vi "Marvin.vi"() -> ()   [LabVIEW 2017]
uses:
  Marvin ATP Remake 1.5.18/PCAN_Driver/ControlCAN.llb/CAN Channel.ctl
  Marvin ATP Remake 6.5.18 - Copy/PCAN_Driver/ControlCAN.llb/DevType.ctl
  Marvin ATP Remake 6.5.18/PCAN_Driver/ControlCAN.llb/VCI_INIT_CONFIG.ctl
  Marvin ATP Remake 6.5.18/PCAN_Driver/ControlCAN.llb/InitFlag.ctl
  Marvin ATP Remake 6.5.18/PCAN_Driver/ControlCAN.llb/Fliter.ctl
  Marvin ATP Remake 6.5.18/PCAN_Driver/ControlCAN.llb/Mode.ctl
  <vilib>/Utility/miscctls.llb/LVMinMaxIncTypeDef.ctl
  PCAN_Driver/ControlCAN.llb/VCI_CAN_OBJ.ctl
  PCAN_Driver/ControlCAN.lvlib
panel:
  in  "Clear Data Array":bool
  in  "PlayPause Data Array":bool
  out "CAN Data":cluster{"Frame Data":u64, "Frame ID":u32}[](array[cluster]) {"Frame ID" format="%.0x"; "Frame Data" format="%016x"}
  out "Waveform Chart":dbl[](graph)
  in  "Help Button":bool
  in  "Clear Monitor":bool
  out "Array":u64[][](array[numeric]) format="%016x"
  out "Ambient Over temp":bool
  out "Ambient Sensor temp":bool
  out "Ambient Temperature":dbl
  in  "Motor Over Temp":bool
  in  "Speed control":bool
  out "Unit Adress":string
  in  "Serial Send":bool
  in  "Index":u16(ring) items=["1"=1, "2"=2, "3"=3]
  out "read buffer":string
  in  "SetGet":enum16{"Get", "Set"}(ring)
  in  "Function":T1(ring)
  in  "Value":dbl
  in  "Value 1/2":enum16{"1", "2"}(ring)
  out "Msg Count":u32
  in  "Param to Set":u16(ring) items=["EBAY 5F"=95, "AHU 3F"=63, "AHU 2F"=47]
  out "UUT":u8
  out "Horizontal Progress Bar":i32(slide) min=0 max=48 scale=0.0..50.0
  in  "Set Param.":bool
  in  "Serial Monitor":bool caption="Graph Button"
  in  "Serial Com":bool
  in  "VISA resource name":refnum<visa-resource-name>="COM6"
  out "Serial Status":bool
  in  "Graph Button":bool
  in  "Refresh Button":bool
  out "Data Send":u64 format="%016x"
  in  "Motor Speed RPM":u16
  out "Under voltage/Over voltage":bool
  out "Speed error":bool
  out "Derated drive temp":bool
  out "Motor Over temperature":bool
  out "Commutation err":bool
  out "Motor Sensor temp Fauilre":bool
  out "Drive Over temperature":bool
  out "Drive Sensor temp Failure":bool
  out "Motor Phase Current RMS":dbl
  out "ECS State":u16
  out "Motor Speed RPM":dbl
  out "Motor Stator Temp.":dbl
  out "Power transistor Heat sink Temp.":dbl
  out "DC Current":dbl
  out "DC Voltage":dbl
  in  "Can Send":bool
  in  "Stop":bool
  out "Config_CANAT":T8 {"DevType" items=["USB-CAN"=3, "USB-CAN2"=4]; "CanIndex" items=["通道1", "通道2"]; "VCI_INIT_CONFIG"."Fliter" items=["接收所有类型"=3, "只接收标准帧"=4, "只接收扩展帧"=7]; "VCI_INIT_CONFIG"."Mode" items=["正常工作", "自测模式（环回）", "仅侦听模式"]; "VCI_INIT_CONFIG"."InitFlag" items=["使用Flash参数", "使用界面设置参数"]}
  in  "Channel 2":T3 caption="Channel" items=["Channel 1", "Channel 2"]
  out "CAN Status":bool
  out "Driver Version":string
  out "Hall Sensor Fault":bool
  out "Motor Phase Current":u16
  in  "Motor Phase Current":u16
  # "ver 1.7"
  # "Marvin"
  # "REDLER TECHNOLOGIES LTD"
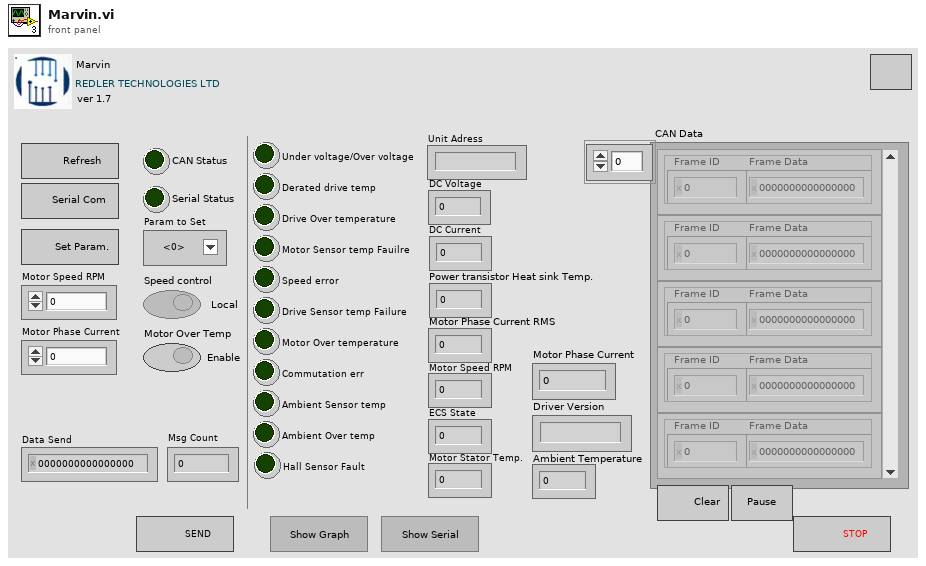
[diagram p1: front panel]
types:
  T1 = enum16{"Enable Conf. EP=1", "Serial Number", "Temperature", "Unit Adress", "Calibration", "Velocity", "Version"}
  T2 = typedef "ControlCAN.lvlib/DevType.ctl" = u32
  T3 = typedef "ControlCAN.lvlib/CAN Channel.ctl" = u32
  T4 = typedef "ControlCAN.lvlib/VCI_INIT_CONFIG.ctl" = cluster{"AccCode":u32, "AccMask":u32, "InitFlag":T5, "Fliter":T6, "Timing0":u8, "Timing1":u8, "Mode":T7}
  T5 = typedef "ControlCAN.lvlib/InitFlag.ctl" = u32
  T6 = typedef "ControlCAN.lvlib/Fliter.ctl" = u8
  T7 = typedef "ControlCAN.lvlib/Mode.ctl" = u8
  T8 = cluster{"DevType":T2, "DevIndex":u32, "CanIndex":T3, "VCI_INIT_CONFIG":T4}
  T9 = cluster{"ID":u32, "MSGTYPE":u8, "LEN":u8, "aDATA":u8[]}[]
  T10 = cluster{"ID":u32, "MSGTYPE":u8, "LEN":u8, "aDATA":u8[]}
  T11 = enum8{"Enabled", "Disabled", "Disabled and Grayed Out"}
  T12 = typedef "LVMinMaxIncTypeDef.ctl" = cluster{"Minimum":dbl, "Maximum":dbl, "Increment":dbl}
  T13 = enum32{"Invalid", "Standard", "Closed", "Hidden", "Minimized", "Maximized"}
  T14 = typedef "ControlCAN.lvlib/VCI_CAN_OBJ.ctl" = cluster{"ID":u32, "TimeStamp":u32, "TimeFlag":u8, "SendType":u8, "RemoteFlag":u8, "ExternFlag":u8, "DataLen":u8, "Data":u8[], "Reserved":u8[]}
  T15 = cluster{"Type":enum16{"接收", "发送"}, "Channel":T3, "Time":timestamp, "VCI_CAN_OBJ":T14}[]
  T16 = cluster{"Type":enum16{"接收", "发送"}, "Channel":T3, "Time":timestamp, "VCI_CAN_OBJ":T14}
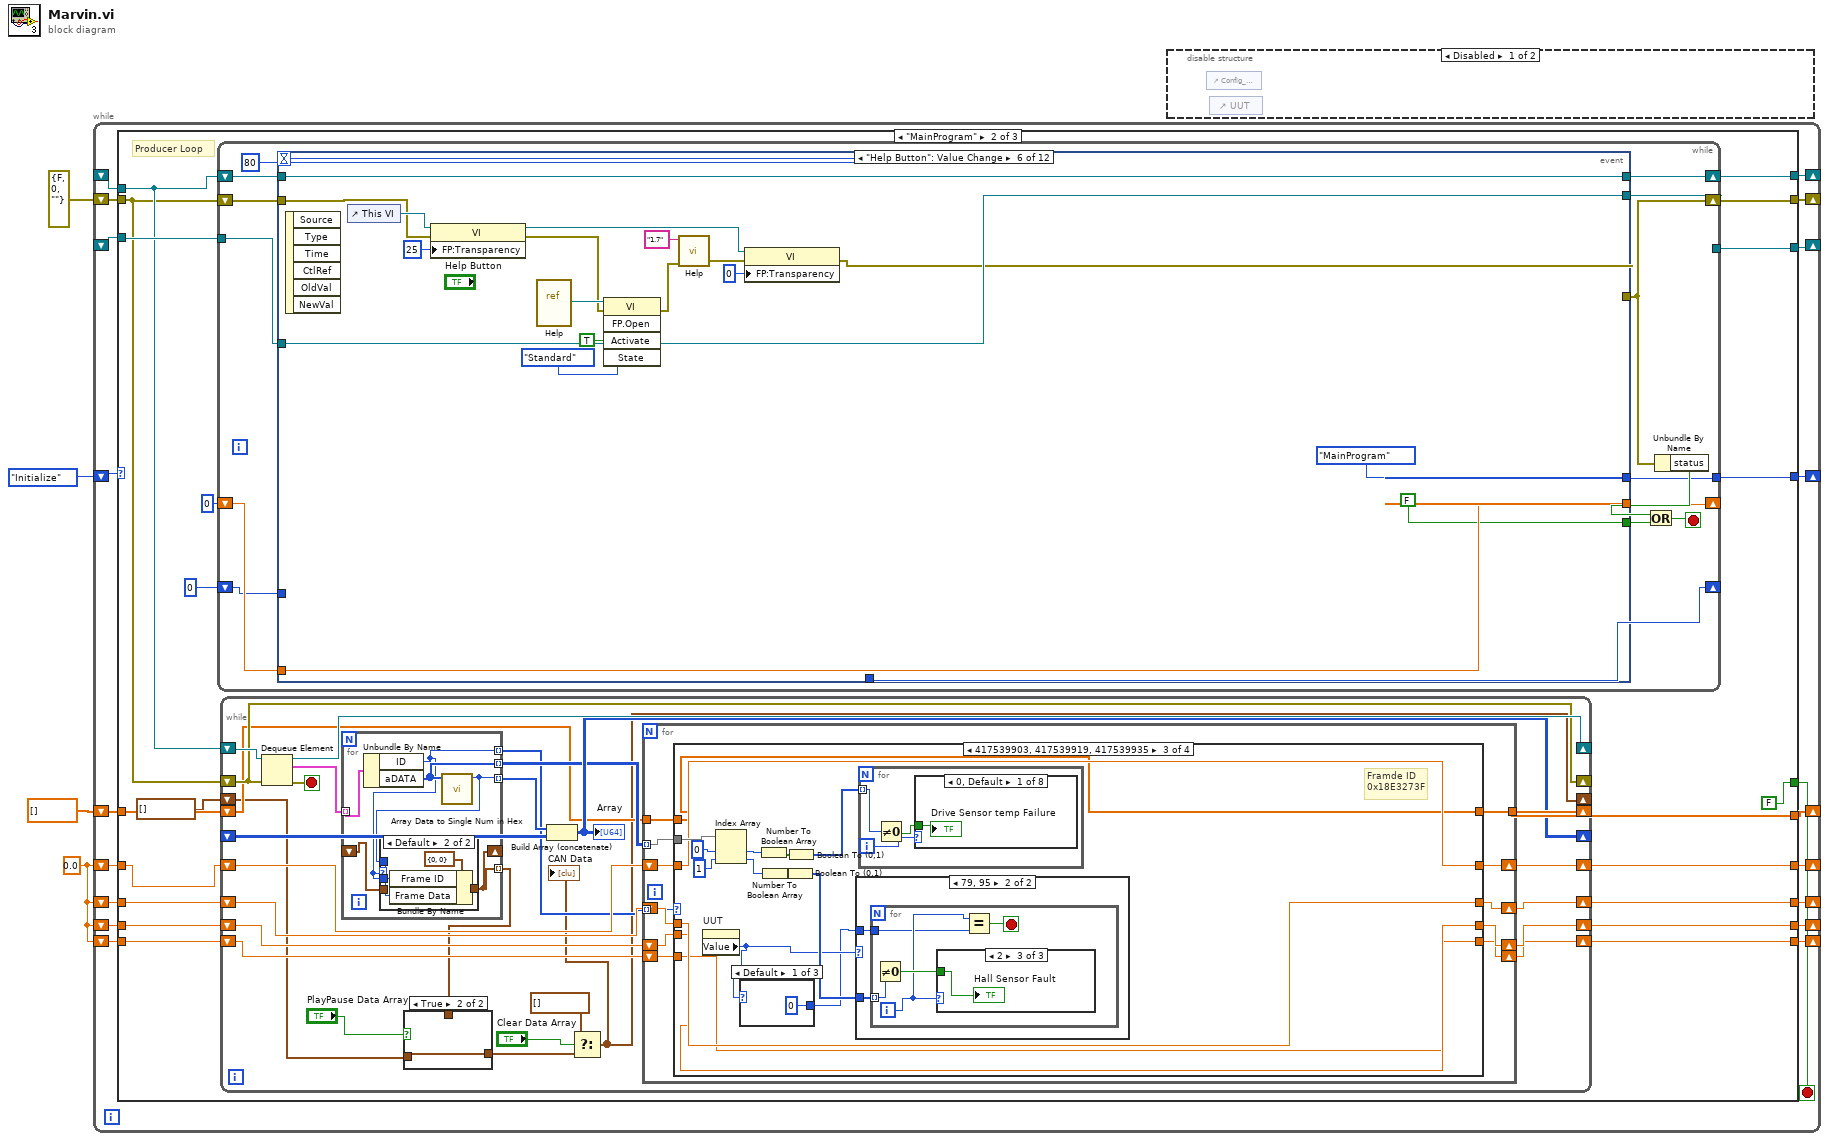
[diagram p0: block diagram]
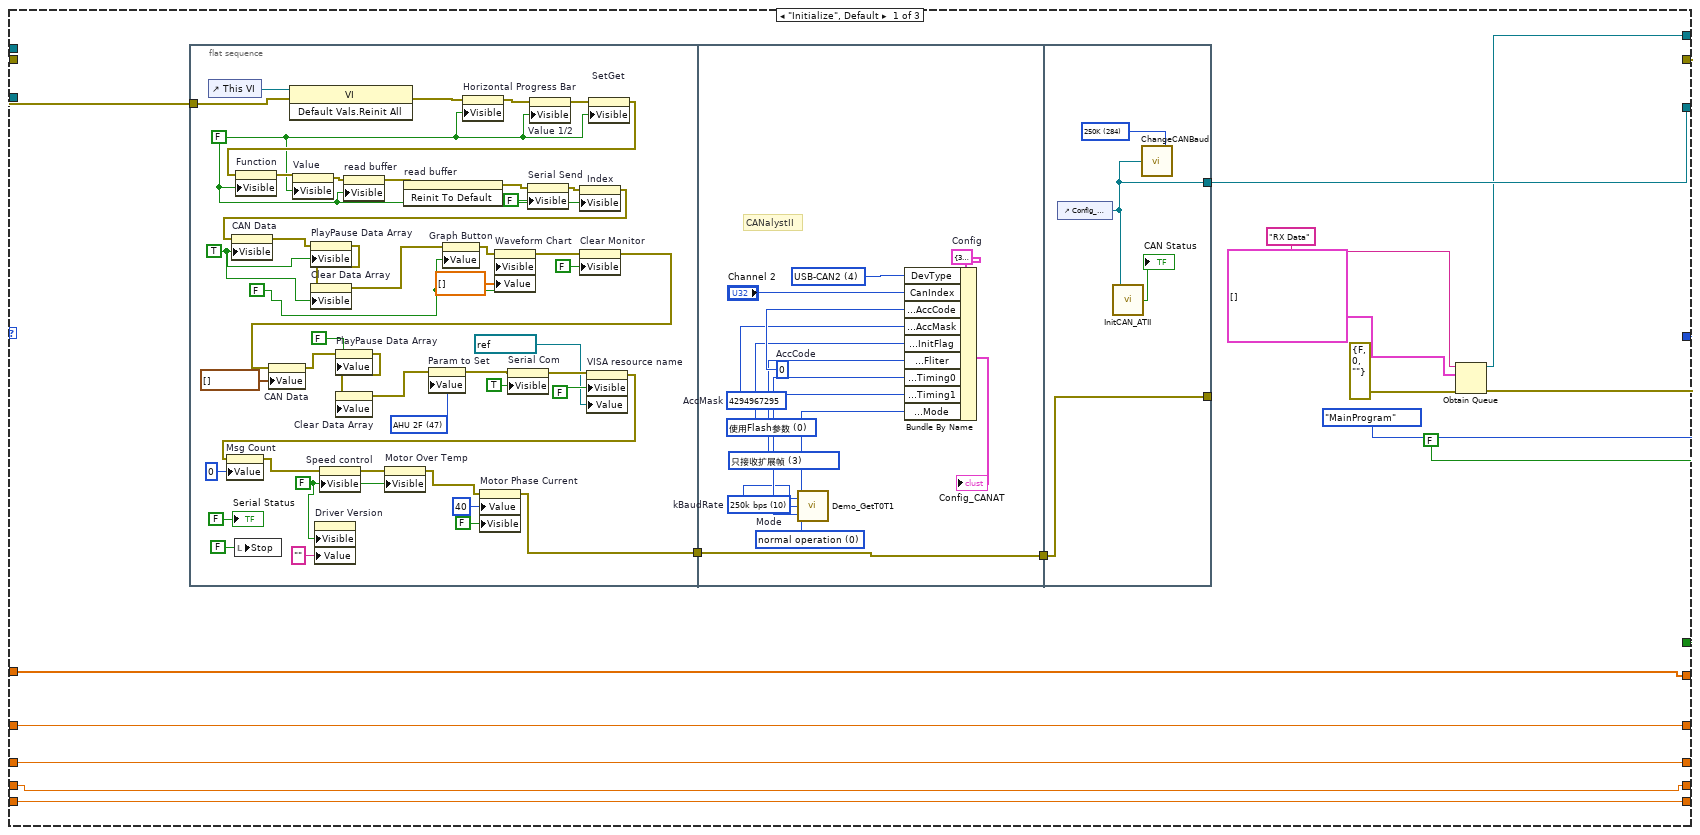
[diagram p3: hidden frame]
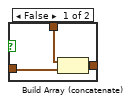
[diagram p4: hidden frame]
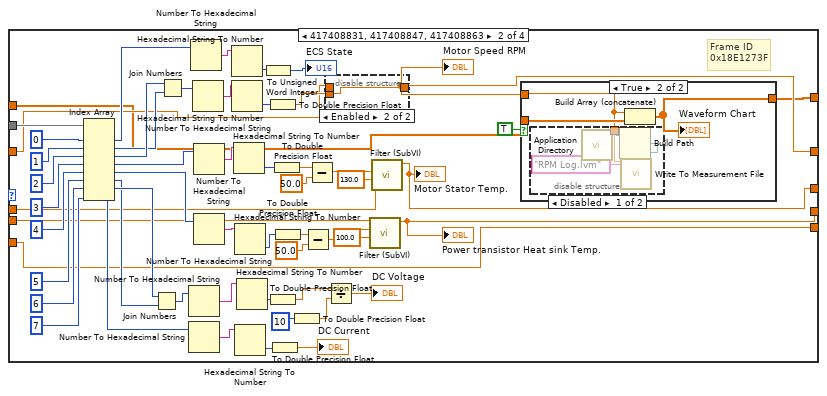
[diagram p6: hidden frame]
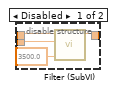
[diagram p7: hidden frame]
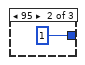
[diagram p10: hidden frame]
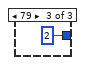
[diagram p11: hidden frame]
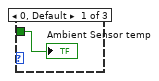
[diagram p13: hidden frame]
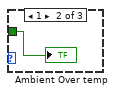
[diagram p14: hidden frame]
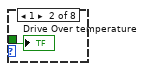
[diagram p15: hidden frame]
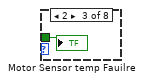
[diagram p16: hidden frame]
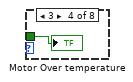
[diagram p17: hidden frame]
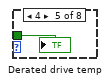
[diagram p18: hidden frame]
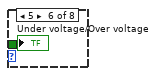
[diagram p19: hidden frame]
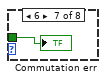
[diagram p20: hidden frame]
diagram:
  w2 = 0.0
  n1 = while {
    shift-right: [w18] -> _
    shift-left: enum16{"Stop", "MainProgram", "Initialize"}."Initialize" -> [w23]
    shift-right: [w22] -> _
    shift-left: _ -> [w21]
    shift-right: [w20] -> _
    shift-left: _ -> [w17]
    shift-right: [w19] -> _
    shift-left: errorcluster {"status"=FALSE, "code"=0, "source"=""} ("error out") -> [w16]
    shift-right: [w10] -> _
    shift-left: w2 -> [w14]
    shift-right: [w7] -> _
    shift-left: w2 -> [w11]
    shift-right: [w8] -> _
    shift-left: w2 -> [w12]
    shift-right: [w9] -> _
    shift-left: w2 -> [w13]
    shift-right: [w5] -> _
    shift-left: dbl[] [] -> [w6]
    stop <- w15 stop-if-true
    n2 = case shown="\"MainProgram\"" w23 {
      tunnel: [w39 w121 w1061] -> w22
      tunnel: w21 -> [_ w124 w1061]
      tunnel: [w35 w123 w1062] -> w20
      tunnel: [w34 w122 w1063] -> w19
      tunnel: [enum16{"Stop", "MainProgram", "Initialize"}."MainProgram" w120 enum16{"Stop", "MainProgram", "Initialize"}."Stop"] -> w18
      tunnel: w17 -> [_ w119 w1062]
      tunnel: w16 -> [w32 w118 w1064]
      tunnel: [FALSE ("Stop") FALSE ("Stop") w1060] -> w15
      tunnel: w14 -> [w28 w109 w1058]
      tunnel: w13 -> [w27 w108 w1057]
      tunnel: w12 -> [w26 w107 w1056]
      tunnel: w11 -> [w25 w106 w1055]
      tunnel: [w28 w115 w1058] -> w10
      tunnel: [w27 w114 w1057] -> w9
      tunnel: [w26 w113 w1056] -> w8
      tunnel: [w25 w112 w1055] -> w7
      tunnel: w6 -> [w24 w111 w1054]
      tunnel: [w24 w110 w1054] -> w5
      frame "Initialize", Default {
        n3 = flat-sequence {
          tunnel: w32 -> [w68]
          tunnel: [w42] -> w30
          tunnel: [w87] -> w31
          tunnel: w30 -> [w87]
          tunnel: [w101] -> w39
          tunnel: w31 -> [w100]
          tunnel: [w100] -> _
          frame #0 {
            w51 = FALSE ("PlayPause Data Array")
            w45 = FALSE ("Visible")
            w78 = u16 47 items=["EBAY 5F"=95, "AHU 3F"=63, "AHU 2F"=47] ("Param to Set")
            w46 = TRUE ("Visible")
            w62 = FALSE ("Visible")
            w50 = FALSE ("Graph Button")
            n4 = control-ref of="This VI"() -> (w86:refnum<vi>)
            n5 = local write "Stop"(FALSE ("Stop")) -> ()
            n6 = invoke class="VI" method="Default Vals.Reinit All"(reference=w86, error in=w68) -> (error out=w67:errorcluster)  [unwired: 1 in, 2 out]
            n7 = property on="Driver Version" class="Str"("Visible"=w45, "Value"="" ("Driver Version")) -> ()  [unwired: 2 in, 2 out]
            n8 = property on="Horizontal Progress Bar" class="Slide (strict)"(error in=w67, "Visible"=w62) -> (error out=w76:errorcluster)  [unwired: 1 in, 1 out]
            n9 = property on="Value 1/2" class="Enum (strict)"(error in=w76, "Visible"=w62) -> (error out=w75:errorcluster)  [unwired: 1 in, 1 out]
            n10 = property on="SetGet" class="Enum (strict)"(error in=w75, "Visible"=w62) -> (error out=w74:errorcluster)  [unwired: 1 in, 1 out]
            n11 = property on="Function" class="Enum (strict)"(error in=w74, "Visible"=w62) -> (error out=w73:errorcluster)  [unwired: 1 in, 1 out]
            n12 = property on="Value" class="DigNum (strict)"(error in=w73, "Visible"=w62) -> (error out=w72:errorcluster)  [unwired: 1 in, 1 out]
            n13 = property on="read buffer" class="Str"(error in=w72, "Visible"=w62) -> (error out=w64:errorcluster)  [unwired: 1 in, 1 out]
            n14 = invoke on="read buffer" class="Str" method="Reinit To Default"(error in=w64) -> (error out=w63:errorcluster)  [unwired: 2 in, 2 out]
            n15 = property on="Serial Send" class="Bool (strict)"(error in=w63, "Visible"=FALSE) -> (error out=w71:errorcluster)  [unwired: 1 in, 1 out]
            n16 = property on="Index" class="Ring (strict)"(error in=w71, "Visible"=w62) -> (error out=w57:errorcluster)  [unwired: 1 in, 1 out]
            n17 = property on="CAN Data" class="Arr (strict)"(error in=w57, "Visible"=w46) -> (error out=w49:errorcluster)  [unwired: 1 in, 1 out]
            n18 = property on="PlayPause Data Array" class="Bool (strict)"(error in=w49, "Visible"=w46) -> (error out=w48:errorcluster)  [unwired: 1 in, 1 out]
            n19 = property on="Clear Data Array" class="Bool (strict)"(error in=w48, "Visible"=w46) -> (error out=w47:errorcluster)  [unwired: 1 in, 1 out]
            n20 = property on="Graph Button" class="Bool (strict)"(error in=w47, "Value"=w50) -> (error out=w60:errorcluster)  [unwired: 1 in, 1 out]
            n21 = property on="Waveform Chart" class="WFChart (strict)"(error in=w60, "Visible"=w50, "Value"=dbl[] [] ("Waveform Chart")) -> (error out=w59:errorcluster)  [unwired: 1 in, 1 out]
            n22 = property on="Clear Monitor" class="Bool"(error in=w59, "Visible"=FALSE) -> (error out=w56:errorcluster)  [unwired: 1 in, 1 out]
            n23 = property on="CAN Data" class="Arr (strict)"(error in=w56, "Value"=cluster{"Frame Data":u64, "Frame ID":u32}[] [] ("CAN Data")) -> (error out=w54:errorcluster)  [unwired: 1 in, 1 out]
            n24 = property on="PlayPause Data Array" class="Bool (strict)"(error in=w54, "Value"=w51) -> (error out=w53:errorcluster)  [unwired: 1 in, 1 out]
            n25 = property on="Clear Data Array" class="Bool (strict)"(error in=w53, "Value"=w51) -> (error out=w52:errorcluster)  [unwired: 1 in, 1 out]
            n26 = property on="Param to Set" class="Ring (strict)"(error in=w52, "Value"=w78) -> (error out=w70:errorcluster)  [unwired: 1 in, 1 out]
            n27 = property on="Serial Com" class="Bool"(error in=w70, "Visible"=TRUE) -> (error out=w83:errorcluster)  [unwired: 1 in, 1 out]
            n28 = property on="VISA resource name" class="VISAName"(error in=w83, "Visible"=FALSE, "Value"=refnum<visa-resource-name> "COM1" ("VISA resource name")) -> (error out=w69:errorcluster)  [unwired: 1 in, 1 out]
            n29 = property on="Msg Count" class="DigNum (strict)"(error in=w69, "Value"=u32 0 ("Msg Count")) -> (error out=w66:errorcluster)  [unwired: 1 in, 1 out]
            n30 = property on="Speed control" class="Bool (strict)"(error in=w66, "Visible"=w45) -> (error out=w65:errorcluster)  [unwired: 1 in, 1 out]
            n31 = property on="Motor Over Temp" class="Bool (strict)"(error in=w65, "Visible"=w45) -> (error out=w43:errorcluster)  [unwired: 1 in, 1 out]
            n32 = property on="Motor Phase Current" class="DigNum (strict)"(error in=w43, "Value"=u16 40 ("Motor Phase Current"), "Visible"=FALSE) -> (error out=w42:errorcluster)  [unwired: 1 in, 1 out]
            "Serial Status" <- FALSE ("Serial Status")
          }
          frame #1 {
            w91 = u32 4294967295  # AccMask
            w90 = T5 0 items=["使用Flash参数", "使用界面设置参数"] ("InitFlag")
            w88 = T7 0 items=["normal operation", "Listen-only mode", "test mode"]  # Mode
            w89 = T6 3 items=["接收所有类型"=1, "只接收标准帧"=2, "只接收扩展帧"=3] ("Fliter")
            w95 = u8 10 items=["5k bps"=1, "10k bps"=2, "20k bps"=3, "40k bps"=4, "50k bps"=5, "80k bps"=6, "100k bps"=7, "125k bps"=8, "200k bps"=9, "250k bps"=10, "400k bps"=11, "500k bps"=12, "666k bps"=13, "800k bps"=14, "1000k bps"=15, "33.33k bps"=16, "66.66k bps"=17, "83.33k bps"=18]  # kBaudRate
            w92 = u32 0  # AccCode
            w93 = T2 4 items=["USB-CAN"=3, "USB-CAN2"=4] ("DevType")
            w94 = T8 {"DevType"=3, "DevIndex"=0, "CanIndex"=0, "VCI_INIT_CONFIG"={"AccCode"=0, "AccMask"=0, "InitFlag"=1, "Fliter"=7, "Timing0"=0, "Timing1"=0, "Mode"=0}}  # Config
            # "CANalystII"
            n33 = call "Demo_GetT0T1.vi"("kBaudRate"=w95) -> ("Timing0"=w97:u8, "Timing1"=w98:u8)
            n34 = Bundle By Name(cluster=w94, "DevType"=w93, "CanIndex"="Channel 2", "VCI_INIT_CONFIG.AccCode"=w92, "VCI_INIT_CONFIG.AccMask"=w91, "VCI_INIT_CONFIG.InitFlag"=w90, "VCI_INIT_CONFIG.Fliter"=w89, "VCI_INIT_CONFIG.Timing0"=w97, "VCI_INIT_CONFIG.Timing1"=w98, "VCI_INIT_CONFIG.Mode"=w88) -> (→"Config_CANAT":T8)
          }
          frame #2 {
            w102 = u16 284 items=["1M"=20, "500K"=28, "250K"=284, "125K"=796, "100K"=17199, "50K"=18223, "20K"=21295, "10K"=26415, "5K"=32639] ("baud in")
            n35 = control-ref of="Config_CANAT"() -> (w101:refnum<vi>)
            n36 = call "InitCAN_ATII.vi"("Config"=w101) -> ("Sts"=→"CAN Status":bool)
            n37 = call "ChangeCANBaud.vi"("baud in"=w102, "reference"=w101) -> ()
          }
        }
        n38 = Obtain Queue(name (unnamed)="RX Data", element data type=T9 [], error in (no error)=errorcluster {"status"=FALSE, "code"=0, "source"=""}) -> (queue out=w35:refnum<queue>, error out=w34:errorcluster)  [unwired: 2 in, 1 out]
      }
      frame "MainProgram" {
        # "Producer Loop"
        n39 = while {
          shift-right: [w330] -> w122
          shift-left: w118 -> [w332]
          shift-right: [w331] -> w123
          shift-left: w119 -> [w333]
          tunnel: w124 -> [w334]
          tunnel: [w327] -> w121
          tunnel: [w326] -> w120
          shift-right: [w324] -> _
          shift-left: 0 -> [w325]
          shift-right: [w322] -> _
          shift-left: 0 -> [w323]
          stop <- w335 stop-if-true
          n40 = event shown="[5] \"Help Button\": Value Change" {
            selector: _ -> [_ _ _ _ _ _ _ _ _ _ _ _]
            dyn-events: _ -> [_ _ _ _ _ _ _ _ _ _ _ _]
            timeout: 80 ("Numeric") -> [_ _ _ _ _ _ _ _ _ _ _ _]
            tunnel: w334 -> [w356 w434 w453 w520 w775 w873 w903 w994 w1014 w1031 w1046 w1052]
            tunnel: w333 -> [w353 w435 w456 w521 w774 w874 w924 w995 w1013 w1032 w1043 w1049]
            tunnel: w332 -> [w338 w433 w451 w508 w767 w866 w923 w974 w1009 w1024 w1042 w1050]
            tunnel: [w351 w435 w456 w521 w774 w874 w924 w995 w1013 w1032 w1041 w1049] -> w331
            tunnel: [w350 w428 w452 w513 w763 w863 w923 w981 w1006 w1022 w1039 w1048] -> w330
            tunnel: [FALSE ("Stop") FALSE ("Stop") FALSE ("Stop") FALSE ("Stop") FALSE ("Stop") FALSE ("Stop") FALSE ("Stop") FALSE ("Stop") FALSE ("Stop") FALSE ("Stop") TRUE ("Stop") TRUE ("Stop")] -> w328
            tunnel: [w349 w434 w453 w520 w775 w873 w903 w994 w1014 w1031 w1046 w1052] -> w327
            tunnel: [enum16{"Stop", "MainProgram", "Initialize"}."MainProgram" enum16{"Stop", "MainProgram", "Initialize"}."MainProgram" enum16{"Stop", "MainProgram", "Initialize"}."MainProgram" enum16{"Stop", "MainProgram", "Initialize"}."MainProgram" enum16{"Stop", "MainProgram", "Initialize"}."MainProgram" enum16{"Stop", "MainProgram", "Initialize"}."MainProgram" enum16{"Stop", "MainProgram", "Initialize"}."MainProgram" enum16{"Stop", "MainProgram", "Initialize"}."MainProgram" enum16{"Stop", "MainProgram", "Initialize"}."MainProgram" enum16{"Stop", "MainProgram", "Initialize"}."MainProgram" enum16{"Stop", "MainProgram", "Initialize"}."Stop" enum16{"Stop", "MainProgram", "Initialize"}."Initialize"] -> w326
            tunnel: w325 -> [w345 w438 w449 w509 w765 w877 w889 w990 w1005 w1020 w1038 w1047]
            tunnel: [w344 w438 w449 w509 w765 w877 w889 w990 w1005 w1020 w1038 w1047] -> w324
            tunnel: w323 -> [w337 _ _ _ _ _ _ _ _ _ _ _]
            tunnel: [w337 _ _ _ _ _ _ _ _ _ _ _] -> w322
            event Timeout {
              n41 = event-data() -> ()  [unwired: 1 in, 3 out]
              n42 = property class="Clust (strict)"(reference=w356) -> (reference out=w349:refnum<vi>, "Value"=w357:T8)  [unwired: 1 in, 1 out]
              n43 = property on="Speed control" class="Bool (strict)"(error in=w338) -> ("Value"=w339:bool)  [unwired: 1 in, 2 out]
              n44 = case shown="True" w339 {
                frame False {
                }
                frame True {
                  n45 = property on="Motor Speed RPM" class="DigNum (strict)"() -> ("Value"=w363:u16)  [unwired: 2 in, 2 out]
                  n46 = control-ref of="Config_CANAT"() -> (w362:refnum<vi>)
                  n47 = control-ref of="UUT"() -> (w361:refnum<vi>)
                  n48 = call "CANSendMotorSpeed.vi"("Remote"=TRUE, "Motor Speed RPM"=w363, "UUT"=w361, "CAN Cluster in"=w362) -> ()  [unwired: 7 in, 1 out]
                }
              }
              n49 = Unbundle By Name(w357) -> ("DevType"=w358:T2, "CanIndex"=w354:T3)
              n50 = property on="Horizontal Progress Bar" class="Slide (strict)"(error in=w338, "Visible"=FALSE) -> (error out=w340:errorcluster)  [unwired: 1 in, 1 out]
              n51 = call "VCI_Receive.vi"("CANIndex"=w354, "DevIndex"=u32 0, "DevType"=w358) -> ("Recieve"=w352:T14[])  [unwired: 3 in, 5 out]
              n52 = Empty Array?(array=w352) -> (empty?=w355:bool)
              n53 = case shown="False" w355 {
                tunnel: w354 -> [w375 _]
                tunnel: w349 -> [w373 _]
                tunnel: w353 -> [w372 w427]
                tunnel: w340 -> [w371 w426]
                tunnel: w352 -> [w376 _]
                tunnel: [w366 w426] -> w350
                tunnel: [w365 w427] -> w351
                tunnel: [w364 0] -> w341
                frame False {
                  n54 = call "Demo_MakeDispBuff.vi"("Channel"=w375, "Type"=enum16{"接收", "发送"}."接收", "OBJs"=w376) -> ("Buffer"=w374:T15)
                  n55 = for {
                    N: 3 -> [_]
                    tunnel: w374 -> [w390]
                    tunnel: w373 -> [w389]
                    tunnel: w372 -> [w380]
                    tunnel: w371 -> [w379]
                    tunnel: [w382] -> w369 mode=indexing
                    tunnel: [w380] -> w368
                    tunnel: [w379] -> w367
                    tunnel: [w378] -> w364
                    i -> [w378]
                    n56 = property class="Clust (strict)"(reference=w389) -> ("Value"=w387:T8)  [unwired: 1 in, 2 out]
                    n57 = Index Array(array=w390, index=w378) -> (element=w383:T16)
                    n58 = Unbundle By Name(w383) -> ("Channel"=w385:T3, "VCI_CAN_OBJ"=w388:T14)  [unwired: 2 out]
                    n59 = Unbundle By Name(w387) -> ("CanIndex"=w386:T3)
                    n60 = Equal?(x=w386, y=w385) -> (x = y?=w384:bool)
                    n61 = case shown="True" w384 {
                      tunnel: w388 -> [_ w406]
                      tunnel: [w391 w402] -> w382
                      tunnel: T10 {"ID"=0, "MSGTYPE"=0, "LEN"=0, "aDATA"=[]} ("Msg") -> [w391 w401]
                      frame False {
                      }
                      frame True {
                        n62 = Unbundle By Name(w406) -> ("ID"=w400:u32, "DataLen"=w405:u8, "Data"=w403:u8[])
                        n63 = Bundle By Name(cluster=w401, "ID"=w400, "MSGTYPE"=u8 0, "LEN"=w405, "aDATA"=w403) -> (w402:T10)
                        n64 = Unbundle By Name(w402) -> ("ID"=w398:u32)
                        n65 = Split Number(x=w398) -> (lo(x)=w399:u16)  [unwired: 1 out]
                        n66 = Split Number(x=w399) -> (lo(x)=w396:u8)  [unwired: 1 out]
                        "UUT" <- w396
                        n67 = case shown="95" w396 {
                          tunnel: ["EBAY 5F" "PUMP 4F" w419 "AHU 3F" "AHU 2F"] -> w395
                          tunnel: [TRUE w416 w420 w421 w423] -> w393
                          tunnel: [TRUE w416 w418 w421 w423] -> w392
                          frame 95 {
                          }
                          frame 79 {
                            w416 = TRUE
                          }
                          frame Default {
                            n68 = property on="Hall Sensor Fault" class="Bool (strict)"() -> ("Visible"=w418:bool)  [unwired: 2 in, 2 out]
                            n69 = property on="Speed control" class="Bool (strict)"() -> ("Visible"=w420:bool)  [unwired: 2 in, 2 out]
                            n70 = property on="Unit Adress" class="Str"() -> ("Value"=w419:string)  [unwired: 2 in, 2 out]
                          }
                          frame 63 {
                            w421 = FALSE
                          }
                          frame 47 {
                            w423 = FALSE
                          }
                        }
                        n71 = Not Equal To 0?(x=w396) -> (x != 0?=w397:bool)
                        n72 = case shown="True" w397 {
                          tunnel: w396 -> [_ w412]
                          tunnel: w395 -> [_ w409]
                          tunnel: [w407 w408] -> w394
                          frame False {
                            n73 = property on="Unit Adress" class="Str"() -> ("Value"=w407:string)  [unwired: 2 in, 2 out]
                          }
                          frame True {
                            n74 = Number To Decimal String(number=w412) -> (decimal integer string=w411:string)  [unwired: 1 in]
                            n75 = call <vilib>:"Space Constant.vi"() -> ("String"=w410:string)
                            n76 = Concatenate Strings(w411, w410, w409) -> (w408:string)
                          }
                        }
                        "Unit Adress" <- w394
                        n77 = property on="Driver Version" class="Str"("Visible"=w393) -> ()  [unwired: 2 in, 2 out]
                        n78 = property on="Hall Sensor Fault" class="Bool (strict)"("Visible"=w392) -> ()  [unwired: 2 in, 2 out]
                        n79 = property on="Motor Phase Current" class="DigNum (strict)"("Visible"=w392) -> ()  [unwired: 2 in, 2 out]
                        n80 = property on="Motor Phase Current" class="DigNum (strict)"("Visible"=w392) -> ()  [unwired: 2 in, 2 out]
                        n81 = property on="Ambient Over temp" class="Bool (strict)"("Visible"=w393) -> ()  [unwired: 2 in, 2 out]
                        n82 = property on="Ambient Sensor temp" class="Bool (strict)"("Visible"=w393) -> ()  [unwired: 2 in, 2 out]
                        n83 = property on="Ambient Temperature" class="DigNum (strict)"("Visible"=w393) -> ()  [unwired: 2 in, 2 out]
                        n84 = property on="Motor Over Temp" class="Bool (strict)"("Visible"=w393) -> ()  [unwired: 2 in, 2 out]
                        n85 = property on="Speed control" class="Bool (strict)"("Visible"=w393) -> ()  [unwired: 2 in, 2 out]
                      }
                    }
                  }
                  n86 = Enqueue Element(queue=w368, element=w369, error in (no error)=w367) -> (queue out=w365:refnum<queue>, error out=w366:errorcluster)  [unwired: 2 out]
                }
                frame True {
                }
              }
              n87 = Divide(x=w341, y=u32 2) -> (x/y=w342:dbl)
              n88 = Add(x=w342, y=w345) -> (x+y=w344:dbl)
              "Msg Count" <- w344
            }
            event "Clear Monitor": Value Change {
              n89 = event-data() -> ()  [unwired: 1 in, 6 out]
              n90 = property on="VISA resource name" class="VISAName"(error in=w433) -> (error out=w432:errorcluster, "Value"=w431:refnum<visa-resource-name>)  [unwired: 1 in, 1 out]
              n91 = disable-structure shown="Enabled" {
                disable-tunnel: w432 -> [w443 w446]
                disable-tunnel: w431 -> [w441 w447]
                disable-tunnel: [w440 ""] -> w430
                disable-tunnel: [w439 w445] -> w429
                frame Disabled {
                  n92 = call "Serial.vi"("error in (no error)"=w443, "Clear Log"=TRUE, "VISA resource name"=w441) -> ("error out"=w439:errorcluster, "read buffer"=w440:string)  [unwired: 7 in]
                }
                frame Enabled {
                  n93 = VISA Flush I/O Buffer(VISA resource name=w447, error in (no error)=w446) -> (error out=w445:errorcluster)  [unwired: 1 in, 1 out]
                }
              }
              n94 = property on="read buffer" class="Str"(error in=w429, "Value"=w430) -> (error out=w428:errorcluster)  [unwired: 1 in, 1 out]
            }
            event "Serial Monitor": Value Change {
              n95 = event-data() -> ()  [unwired: 1 in, 6 out]
              n96 = property on="Serial Status" class="Bool (strict)"(error in=w451) -> (error out=w450:errorcluster, "Value"=w448:bool)  [unwired: 1 in, 1 out]
              n97 = case shown="True" w448 {
                tunnel: w450 -> [w460 w473]
                tunnel: [w458 w478] -> w452
                frame False {
                  n98 = call "Display Message to User3"("error in (no error)"=w460) -> ("error out"=w459:errorcluster)  [unwired: 9 in, 1 out]
                  n99 = property on="Serial Monitor" class="Bool (strict)"(error in=w459, "Value"=FALSE ("Serial Monitor")) -> (error out=w458:errorcluster)  [unwired: 1 in, 1 out]
                }
                frame True {
                  w465 = FALSE ("Visible")
                  w475 = FALSE ("Visible")
                  w476 = u16 1 items=["1"=1, "2"=2, "3"=3] ("Index")
                  n100 = property on="Index" class="Ring (strict)"(error in=w473, "Value"=w476) -> (error out=w472:errorcluster)  [unwired: 1 in, 1 out]
                  n101 = property on="Value 1/2" class="Enum (strict)"(error in=w472, "Visible"=w475) -> (error out=w471:errorcluster)  [unwired: 1 in, 1 out]
                  n102 = property on="Value" class="DigNum (strict)"(error in=w471, "Visible"=w475) -> (error out=w470:errorcluster)  [unwired: 1 in, 1 out]
                  n103 = property on="SetGet" class="Enum (strict)"(error in=w470, "Value"=enum16{"Get", "Set"}."Get" ("SetGet")) -> (error out=w469:errorcluster)  [unwired: 1 in, 1 out]
                  n104 = property on="Serial Send" class="Bool (strict)"(error in=w469, "Visible"=w465) -> (error out=w464:errorcluster)  [unwired: 1 in, 1 out]
                  n105 = property on="Clear Monitor" class="Bool"(error in=w464, "Visible"=w465) -> (error out=w463:errorcluster)  [unwired: 1 in, 1 out]
                  n106 = property on="Function" class="Enum (strict)"(error in=w463, "Value"=T1."Serial Number" ("Function")) -> (error out=w468:errorcluster)  [unwired: 1 in, 1 out]
                  n107 = property on="Index" class="Ring (strict)"(error in=w468, "DisabledEnum"=T11."Disabled and Grayed Out" ("Disabled")) -> (error out=w466:errorcluster)  [unwired: 1 in, 1 out]
                  n108 = case shown="True" "Serial Monitor" {
                    selector: "Serial Monitor" -> [w482 w503]
                    tunnel: w466 -> [w481 w499]
                    tunnel: [w484 w500] -> w478
                    tunnel: [FALSE TRUE] -> w462
                    frame False {
                      n109 = property on="Graph Button" class="Bool (strict)"(error in=w481) -> (error out=w480:errorcluster, "Value"=w479:bool)  [unwired: 1 in, 1 out]
                      n110 = case shown="True" w479 {
                        tunnel: [w488 w493] -> w485
                        tunnel: w480 -> [w490 w496]
                        tunnel: w482 -> [w491 _]
                        frame False {
                          n111 = property on="Waveform Chart" class="WFChart (strict)"(error in=w490, "Visible"=FALSE) -> (error out=w487:errorcluster)  [unwired: 1 in, 1 out]
                          n112 = Not(x=w491) -> (.not. x?=w486:bool)
                          n113 = property on="PlayPause Data Array" class="Bool (strict)"("Visible"=w486) -> ()  [unwired: 2 in, 2 out]
                          n114 = property on="Clear Data Array" class="Bool (strict)"("Visible"=w486) -> ()  [unwired: 2 in, 2 out]
                          n115 = property on="CAN Data" class="Arr (strict)"(error in=w487, "Visible"=w486) -> (error out=w488:errorcluster)  [unwired: 1 in, 1 out]
                        }
                        frame True {
                          w492 = FALSE ("Visible")
                          n116 = property on="Waveform Chart" class="WFChart (strict)"(error in=w496, "Visible"=TRUE) -> (error out=w494:errorcluster)  [unwired: 1 in, 1 out]
                          n117 = property on="PlayPause Data Array" class="Bool (strict)"("Visible"=w492) -> ()  [unwired: 2 in, 2 out]
                          n118 = property on="Clear Data Array" class="Bool (strict)"("Visible"=w492) -> ()  [unwired: 2 in, 2 out]
                          n119 = property on="CAN Data" class="Arr (strict)"(error in=w494, "Visible"=w492) -> (error out=w493:errorcluster)  [unwired: 1 in, 1 out]
                        }
                      }
                      n120 = property on="Serial Monitor" class="Bool (strict)"(error in=w485, "Value"=w482) -> (error out=w484:errorcluster)  [unwired: 1 in, 1 out]
                    }
                    frame True {
                      n121 = Not(x=w503) -> (.not. x?=w497:bool)
                      n122 = property on="PlayPause Data Array" class="Bool (strict)"("Visible"=w497) -> ()  [unwired: 2 in, 2 out]
                      n123 = property on="CAN Data" class="Arr (strict)"(error in=w499, "Visible"=w497) -> (error out=w498:errorcluster)  [unwired: 1 in, 1 out]
                      n124 = property on="Clear Data Array" class="Bool (strict)"("Visible"=w497) -> ()  [unwired: 2 in, 2 out]
                      n125 = property on="Serial Monitor" class="Bool (strict)"(error in=w498, "Value"=w503) -> (error out=w502:errorcluster)  [unwired: 1 in, 1 out]
                      n126 = property on="Graph Button" class="Bool (strict)"(error in=w502, "Value"=w497) -> (error out=w501:errorcluster)  [unwired: 1 in, 1 out]
                      n127 = property on="Waveform Chart" class="WFChart (strict)"(error in=w501, "Visible"=w497) -> (error out=w500:errorcluster)  [unwired: 1 in, 1 out]
                    }
                  }
                  n128 = property on="SetGet" class="Enum (strict)"("Visible"=w462) -> ()  [unwired: 2 in, 2 out]
                  n129 = property on="Index" class="Ring (strict)"("Visible"=w462) -> ()  [unwired: 2 in, 2 out]
                  n130 = property on="Function" class="Enum (strict)"("Visible"=w462) -> ()  [unwired: 2 in, 2 out]
                  n131 = property on="Clear Monitor" class="Bool"("Visible"=w462) -> ()  [unwired: 2 in, 2 out]
                  n132 = property on="Serial Send" class="Bool (strict)"("Visible"=w462) -> ()  [unwired: 2 in, 2 out]
                  n133 = property on="read buffer" class="Str"("Visible"=w462) -> ()  [unwired: 2 in, 2 out]
                }
              }
            }
            event "Serial Send", "Function", "SetGet": Value Change {
              n134 = event-data() -> ()  [unwired: 1 in, 6 out]
              n135 = case shown="\"Enable Conf. EP=1\"" "Function" {
                tunnel: w508 -> [w527 w532 w539 w541 w544 w548 w550 w551]
                tunnel: [w526 w534 w538 w543 w546 w547 w550 w551] -> w506
                frame "Serial Number" {
                  n136 = property on="Index" class="Ring (strict)"(error in=w527, "DisabledEnum"=T11."Disabled and Grayed Out" ("Disabled")) -> (error out=w526:errorcluster)  [unwired: 1 in, 1 out]
                }
                frame "Temperature" {
                  n137 = property on="UUT" class="DigNum (strict)"() -> ("Value"=w529:u8)  [unwired: 2 in, 2 out]
                  n138 = case shown="95" w529 {
                    tunnel: [i32[] [2] ("Disabled Items []") i32[] [3] ("Disabled Items []")] -> w530
                    frame 47, 63, Default {
                    }
                    frame 95 {
                    }
                  }
                  n139 = property on="Index" class="Ring (strict)"(error in=w532, "DisabledEnum"=T11."Enabled" ("Disabled"), "Visible"=TRUE, "Disabled Items []"=w530) -> (error out=w534:errorcluster)  [unwired: 1 in, 1 out]
                }
                frame "Unit Adress" {
                  n140 = property on="Index" class="Ring (strict)"(error in=w539, "DisabledEnum"=T11."Enabled" ("Disabled"), "Visible"=TRUE) -> (error out=w538:errorcluster)  [unwired: 1 in, 1 out]
                }
                frame "Calibration" {
                  n141 = property on="Index" class="Ring (strict)"(error in=w541, "DisabledEnum"=T11."Disabled and Grayed Out" ("Disabled")) -> (error out=w543:errorcluster)  [unwired: 1 in, 1 out]
                }
                frame "Velocity" {
                  n142 = property on="Index" class="Ring (strict)"(error in=w544, "DisabledEnum"=T11."Disabled and Grayed Out" ("Disabled")) -> (error out=w546:errorcluster)  [unwired: 1 in, 1 out]
                }
                frame "Version" {
                  n143 = property on="Index" class="Ring (strict)"(error in=w548, "DisabledEnum"=T11."Disabled and Grayed Out" ("Disabled")) -> (error out=w547:errorcluster)  [unwired: 1 in, 1 out]
                }
                frame "Enable Conf. EP=1" {
                }
                frame Default {
                }
              }
              n144 = property on="VISA resource name" class="VISAName"() -> ("Value"=w522:refnum<visa-resource-name>)  [unwired: 2 in, 2 out]
              n145 = property on="read buffer" class="Str"(error in=w506) -> (error out=w515:errorcluster, "Text.Scroll Position"=w512:u32)  [unwired: 1 in, 1 out]
              n146 = case shown="\"Set\"" "SetGet" {
                tunnel: "Function" -> [w555 w654]
                tunnel: w522 -> [w561 w664]
                tunnel: w515 -> [w558 w653]
                tunnel: "Value" -> [_ w663]
                tunnel: "Value 1/2" -> [_ w661]
                tunnel: "Index" -> [w556 w658]
                tunnel: [w560 w656] -> w514
                tunnel: [w553 w655] -> w519
                tunnel: "Serial Send" -> [w552 w645]
                frame "Get", Default {
                  w559 = FALSE ("Visible")
                  n147 = property on="Value" class="DigNum (strict)"(error in=w558, "Visible"=w559) -> (error out=w557:errorcluster)  [unwired: 1 in, 1 out]
                  n148 = property on="Value 1/2" class="Enum (strict)"(error in=w557, "Visible"=w559) -> (error out=w554:errorcluster)  [unwired: 1 in, 1 out]
                  n149 = case shown="True" w552 {
                    tunnel: w561 -> [_ w572]
                    tunnel: [w562 w567] -> w560
                    tunnel: w556 -> [_ w571]
                    tunnel: w555 -> [_ w570]
                    tunnel: w554 -> [w562 w569]
                    tunnel: [w563 w565] -> w553
                    frame False {
                      n150 = property on="read buffer" class="Str"() -> ("Value"=w563:string)  [unwired: 2 in, 2 out]
                    }
                    frame True {
                      n151 = case shown="\"Serial Number\"" w570 {
                        tunnel: w572 -> [w577 w595 w611 w620 w627 w638 _]
                        tunnel: w569 -> [w575 w586 w601 w615 w625 w636 w643]
                        tunnel: [w580 w596 w612 w621 w631 w639 w643] -> w567
                        tunnel: [w579 w597 w610 w622 w632 w634 "Cannot perform operation.\n" ("read buffer")] -> w566
                        tunnel: w571 -> [_ w590 w603 _ _ _ _]
                        frame "Serial Number" {
                          n152 = property on="Index" class="Ring (strict)"(error in=w575, "DisabledEnum"=T11."Disabled and Grayed Out" ("Disabled")) -> (error out=w574:errorcluster)  [unwired: 1 in, 1 out]
                          n153 = Concatenate Strings("SN" ("string"), "\r\n" ("write buffer")) -> (w578:string)
                          n154 = call "Serial.vi"("error in (no error)"=w574, "Clear Log"=FALSE, "write buffer"=w578, "VISA resource name"=w577) -> ("error out"=w580:errorcluster, "read buffer"=w579:string)  [unwired: 6 in]
                        }
                        frame "Temperature" {
                          n155 = Number To Decimal String(number=w590) -> (decimal integer string=w589:string)  [unwired: 1 in]
                          n156 = property on="Index" class="Ring (strict)"(error in=w586, "DisabledEnum"=T11."Enabled" ("Disabled"), "Visible"=TRUE) -> (error out=w585:errorcluster)  [unwired: 1 in, 1 out]
                          n157 = Concatenate Strings("TA" ("string"), "[", w589, "]", "\r\n" ("write buffer")) -> (w591:string)
                          n158 = call "Serial.vi"("error in (no error)"=w585, "Clear Log"=FALSE, "write buffer"=w591, "VISA resource name"=w595) -> ("error out"=w596:errorcluster, "read buffer"=w597:string)  [unwired: 6 in]
                        }
                        frame "Unit Adress" {
                          n159 = Number To Decimal String(number=w603) -> (decimal integer string=w609:string)  [unwired: 1 in]
                          n160 = property on="Index" class="Ring (strict)"(error in=w601, "DisabledEnum"=T11."Enabled" ("Disabled"), "Visible"=TRUE) -> (error out=w600:errorcluster)  [unwired: 1 in, 1 out]
                          n161 = Concatenate Strings("UA" ("string"), "[", w609, "]", "\r\n" ("write buffer")) -> (w604:string)
                          n162 = call "Serial.vi"("error in (no error)"=w600, "Clear Log"=FALSE, "write buffer"=w604, "VISA resource name"=w611) -> ("error out"=w612:errorcluster, "read buffer"=w610:string)  [unwired: 6 in]
                        }
                        frame "Calibration" {
                          n163 = property on="Index" class="Ring (strict)"(error in=w615, "DisabledEnum"=T11."Disabled and Grayed Out" ("Disabled")) -> (error out=w614:errorcluster)  [unwired: 1 in, 1 out]
                          n164 = Concatenate Strings("CC" ("string"), "\r\n" ("write buffer")) -> (w618:string)
                          n165 = call "Serial.vi"("error in (no error)"=w614, "Clear Log"=FALSE, "write buffer"=w618, "VISA resource name"=w620) -> ("error out"=w621:errorcluster, "read buffer"=w622:string)  [unwired: 6 in]
                        }
                        frame "Velocity" {
                          n166 = property on="Index" class="Ring (strict)"(error in=w625, "DisabledEnum"=T11."Disabled and Grayed Out" ("Disabled")) -> (error out=w624:errorcluster)  [unwired: 1 in, 1 out]
                          n167 = Concatenate Strings("VC" ("string"), "\r\n" ("write buffer")) -> (w628:string)
                          n168 = call "Serial.vi"("error in (no error)"=w624, "Clear Log"=FALSE, "write buffer"=w628, "VISA resource name"=w627) -> ("error out"=w631:errorcluster, "read buffer"=w632:string)  [unwired: 6 in]
                        }
                        frame "Version" {
                          n169 = Concatenate Strings("VR" ("string"), "\r\n" ("write buffer")) -> (w640:string)
                          n170 = property on="Index" class="Ring (strict)"(error in=w636, "DisabledEnum"=T11."Disabled and Grayed Out" ("Disabled")) -> (error out=w635:errorcluster)  [unwired: 1 in, 1 out]
                          n171 = call "Serial.vi"("error in (no error)"=w635, "Clear Log"=FALSE, "write buffer"=w640, "VISA resource name"=w638) -> ("error out"=w639:errorcluster, "read buffer"=w634:string)  [unwired: 6 in]
                        }
                        frame Default {
                        }
                      }
                      n172 = property on="Serial Send" class="Bool (strict)"(error in=w567, "Value"=FALSE ("Serial Send")) -> ()  [unwired: 1 in, 2 out]
                      n173 = property on="read buffer" class="Str"() -> ("Value"=w564:string)  [unwired: 2 in, 2 out]
                      n174 = Concatenate Strings(w564, w566) -> (w565:string)
                    }
                  }
                }
                frame "Set" {
                  n175 = To Unsigned Long Integer(number=w663) -> (unsigned 32bit integer=w659:u32)
                  n176 = Number To Decimal String(number=w658) -> (decimal integer string=w657:string)  [unwired: 1 in]
                  n177 = Number To Decimal String(number=w661) -> (decimal integer string=w660:string)  [unwired: 1 in]
                  n178 = case shown="Default" w654 {
                    tunnel: w653 -> [w738 w742 w746 w750 w754 w758 w760 w762]
                    tunnel: [FALSE TRUE TRUE FALSE FALSE FALSE w759 w761] -> w651
                    tunnel: [TRUE TRUE TRUE FALSE TRUE FALSE w759 w761] -> w650
                    tunnel: [FALSE FALSE FALSE TRUE FALSE FALSE w759 w761] -> w649
                    tunnel: [w738 w742 w746 w750 w754 w758 w760 w762] -> w647
                    frame "Serial Number" {
                    }
                    frame "Temperature" {
                    }
                    frame "Unit Adress" {
                    }
                    frame "Calibration" {
                    }
                    frame "Velocity" {
                    }
                    frame "Version" {
                    }
                    frame "Enable Conf. EP=1" {
                      w759 = FALSE
                    }
                    frame Default {
                      w761 = FALSE
                    }
                  }
                  n179 = Number To Decimal String(number=w659) -> (decimal integer string=w662:string)  [unwired: 1 in]
                  n180 = property on="Index" class="Ring (strict)"(error in=w647, "Visible"=w651) -> (error out=w652:errorcluster)  [unwired: 1 in, 1 out]
                  n181 = property on="Value" class="DigNum (strict)"(error in=w652, "Visible"=w650) -> (error out=w648:errorcluster)  [unwired: 1 in, 1 out]
                  n182 = property on="Value 1/2" class="Enum (strict)"(error in=w648, "Visible"=w649) -> (error out=w646:errorcluster)  [unwired: 1 in, 1 out]
                  n183 = case shown="True" w645 {
                    tunnel: w664 -> [_ w678]
                    tunnel: w662 -> [_ w677]
                    tunnel: w660 -> [_ w676]
                    tunnel: w659 -> [_ w675]
                    tunnel: w657 -> [_ w674]
                    tunnel: [w665 w673] -> w656
                    tunnel: [w666 w672] -> w655
                    tunnel: w654 -> [_ w670]
                    tunnel: w646 -> [w665 w669]
                    frame False {
                      n184 = property on="read buffer" class="Str"() -> ("Value"=w666:string)  [unwired: 2 in, 2 out]
                    }
                    frame True {
                      n185 = flat-sequence {
                        tunnel: [w682] -> w680
                        tunnel: w669 -> [w682]
                        frame #0 {
                          n186 = Wait (ms)(milliseconds to wait=u32 50) -> ()  [unwired: 1 out]
                        }
                      }
                      n187 = case shown="\"Velocity\"" w670 {
                        tunnel: [w685 w691 w700 w708 w726 "EP=1\r\n" ("write buffer") "Cannot perform operation.\n" ("read buffer")] -> w671
                        tunnel: w680 -> [w684 w690 w699 w713 w717 w729 w731]
                        tunnel: [w684 w690 w699 w713 w714 w729 w731] -> w679
                        tunnel: w677 -> [w686 w692 w705 _ _ _ _]
                        tunnel: w676 -> [_ _ _ w709 _ _ _]
                        tunnel: w675 -> [_ _ _ _ w718 _ _]
                        tunnel: w674 -> [_ w693 w703 _ _ _ _]
                        frame "Serial Number" {
                          n188 = Concatenate Strings("SN" ("write buffer"), "=" ("string"), w686, "\r\n" ("write buffer")) -> (w685:string)
                        }
                        frame "Temperature" {
                          n189 = Concatenate Strings("TA" ("string"), "[", w693, "]", "=" ("string"), w692, "\r\n" ("write buffer")) -> (w691:string)
                        }
                        frame "Unit Adress" {
                          n190 = Concatenate Strings("UA" ("string"), "[", w703, "]", "=" ("string"), w705, "\r\n" ("write buffer")) -> (w700:string)
                        }
                        frame "Calibration" {
                          n191 = Concatenate Strings("CC" ("string"), "=" ("string"), w709, "\r\n" ("write buffer")) -> (w708:string)
                        }
                        frame "Velocity" {
                          n192 = In Range and Coerce(upper limit=u16 18001, x=w718, lower limit=u16 0) -> (coerced(x)=w724:u32, In Range?=w722:bool)
                          n193 = Not(x=w722) -> (.not. x?=w723:bool)
                          n194 = Select(t=w724, s=w722, f=u16 0) -> (s? t:f=w716:u32)
                          n195 = Number To Decimal String(number=w716) -> (decimal integer string=w715:string)  [unwired: 1 in]
                          n196 = Concatenate Strings("VC" ("write buffer"), "=" ("string"), w715, "\r\n" ("write buffer")) -> (w726:string)
                          n197 = call "Display Message to User2"("error in (no error)"=w717, "Enable"=w723) -> ("error out"=w714:errorcluster)  [unwired: 8 in, 1 out]
                        }
                        frame "Enable Conf. EP=1" {
                        }
                        frame Default {
                        }
                      }
                      n198 = property on="read buffer" class="Str"() -> ("Value"=w667:string)  [unwired: 2 in, 2 out]
                      n199 = VISA Write(VISA resource name=w678, write buffer=w671, error in (no error)=w679) -> (error out=w681:errorcluster)  [unwired: 2 out]
                      n200 = Concatenate Strings(w667, w671) -> (w672:string)
                      n201 = property on="Serial Send" class="Bool (strict)"("Value"=FALSE ("Serial Send")) -> ()  [unwired: 2 in, 2 out]
                      n202 = flat-sequence {
                        tunnel: w681 -> [w733]
                        tunnel: [w733] -> w673
                        frame #0 {
                          n203 = Wait (ms)(milliseconds to wait=u32 50) -> ()  [unwired: 1 out]
                        }
                      }
                    }
                  }
                }
              }
              "read buffer" <- w519
              n204 = Add(x=u32 5, y=w512) -> (x+y=w511:u32)
              n205 = property on="read buffer" class="Str"(error in=w514, "Text.Scroll Position"=w511) -> (error out=w513:errorcluster)  [unwired: 1 in, 1 out]
            }
            event "Set Param.": Value Change {
              n206 = event-data() -> ()  [unwired: 1 in, 6 out]
              n207 = property on="Serial Status" class="Bool (strict)"(error in=w767) -> (error out=w766:errorcluster, "Value"=w771:bool)  [unwired: 1 in, 1 out]
              n208 = case shown="True" w771 {
                tunnel: w766 -> [w783 w796]
                tunnel: [w782 w792] -> w769
                frame False {
                  n209 = call "Display Message to User4"("error in (no error)"=w783) -> ("error out"=w782:errorcluster)  [unwired: 9 in, 1 out]
                }
                frame True {
                  w785 = FALSE ("Visible")
                  n210 = property on="Speed control" class="Bool (strict)"(error in=w796, "Visible"=FALSE) -> (error out=w795:errorcluster)  [unwired: 1 in, 1 out]
                  n211 = case shown="47" "Param to Set" {
                    tunnel: [w849 w853 w857] -> w811
                    tunnel: w795 -> [w848 w852 w856]
                    tunnel: [w848 w852 w856] -> w799
                    frame 95, Default {
                      n212 = call <vilib>:"Application Directory.vi"() -> ("Application Directory"=w851:path)
                      n213 = Build Path(base path=w851, name or relative path="data\\Marvin_EBAY_params_RRPAR000017_95_v0.2.txt") -> (appended path=w849:path)
                    }
                    frame 63 {
                      n214 = call <vilib>:"Application Directory.vi"() -> ("Application Directory"=w855:path)
                      n215 = Build Path(base path=w855, name or relative path="data\\Marvin_AHU_params_RRPAR000016_63_v0.2.txt") -> (appended path=w853:path)
                    }
                    frame 47 {
                      n216 = call <vilib>:"Application Directory.vi"() -> ("Application Directory"=w859:path)
                      n217 = Build Path(base path=w859, name or relative path="data\\Marvin_AHU_params_RRPAR000015_47_v0.2.txt") -> (appended path=w857:path)
                    }
                  }
                  n218 = property on="read buffer" class="Str"(error in=w799, "Visible"=TRUE) -> (error out=w787:errorcluster)  [unwired: 1 in, 1 out]
                  n219 = property on="CAN Data" class="Arr (strict)"(error in=w787, "Visible"=w785) -> (error out=w786:errorcluster)  [unwired: 1 in, 1 out]
                  n220 = property on="PlayPause Data Array" class="Bool (strict)"("Visible"=w785) -> ()  [unwired: 2 in, 2 out]
                  n221 = property on="Clear Data Array" class="Bool (strict)"("Visible"=w785) -> ()  [unwired: 2 in, 2 out]
                  n222 = property on="Horizontal Progress Bar" class="Slide (strict)"(error in=w786, "Visible"=TRUE, "Value"=u8 0 ("Horizontal Progress Bar")) -> (error out=w794:errorcluster)  [unwired: 1 in, 1 out]
                  n223 = call <vilib>:"Read Characters From File.vi"("file path (dialog if empty)"=w811) -> ("character string"=w812:string)  [unwired: 5 in, 3 out]
                  n224 = while {
                    shift-right: [w840] -> _
                    shift-left: w812 -> [w841]
                    shift-right: [w836] -> w797
                    shift-left: string[] [] -> [w837]
                    tunnel: w794 -> [w829]
                    tunnel: [w829] -> w809
                    stop <- w842 stop-if-true
                    n225 = Match Pattern(string=w841, regular expression="\r\n") -> (before substring=w838:string, after substring=w840:string, offset past match=w839:i32)  [unwired: 1 in, 1 out]
                    n226 = call <vilib>:"Trim Whitespace.vi"("string"=w838) -> ("trimmed string"=w835:string)  [unwired: 1 in]
                    n227 = Equal?(x=w839, y=-1) -> (x = y?=w842:bool)
                    n228 = To Upper Case(1:w835) -> (0:w833:string)
                    n229 = String Length(string=w833) -> (length=w832:i32)
                    n230 = Greater?(x=w832, y=3) -> (0:w830:bool)
                    n231 = case shown="True" w830 {
                      tunnel: w837 -> [w844 w847]
                      tunnel: [w844 w846] -> w836
                      tunnel: w833 -> [_ w845]
                      frame False {
                      }
                      frame True {
                        n232 = Build Array (concatenate)(w847, w845) -> (w846:string[])
                      }
                    }
                  }
                  n233 = property on="VISA resource name" class="VISAName"(error in=w809) -> (error out=w802:errorcluster, "Value"=w791:refnum<visa-resource-name>)  [unwired: 1 in, 1 out]
                  n234 = Build Array (concatenate)(w797, string[] ["MT", "VR", "SN"] ("array")) -> (w806:string[])
                  n235 = Array Size(array=w806) -> (size(s)=w798:i32)
                  n236 = Bundle By Name(cluster=T12 {"Minimum"=0.0, "Maximum"=0.0, "Increment"=0.0} ("Data Entry Limits"), "Minimum"=0.0, "Maximum"=w798) -> (w804:T12)
                  n237 = property on="Horizontal Progress Bar" class="Slide (strict)"(error in=w802, "Data Range"=w804) -> (error out=w790:errorcluster)  [unwired: 1 in, 1 out]
                  n238 = property on="read buffer" class="Str"(error in=w790) -> (error out=w789:errorcluster, "Text.Scroll Position"=w788:u32)  [unwired: 1 in, 1 out]
                  n239 = for {
                    tunnel: w806 -> [w820] mode=indexing
                    tunnel: w791 -> [w826]
                    tunnel: w789 -> [w825]
                    tunnel: [w817] -> w793
                    tunnel: w788 -> [w816]
                    i -> [w815]
                    n240 = Concatenate Strings(w820, "\r\n" ("string")) -> (w818:string)
                    n241 = VISA Write(VISA resource name=w826, write buffer=w818, error in (no error)=w825) -> (error out=w824:errorcluster)  [unwired: 2 out]
                    n242 = flat-sequence {
                      tunnel: w824 -> [w827]
                      tunnel: [w827] -> w817
                      frame #0 {
                        n243 = Wait (ms)(milliseconds to wait=u32 50) -> ()  [unwired: 1 out]
                      }
                    }
                    n244 = Add(x=w816, y=w815) -> (x+y=w814:u32)
                    n245 = feedback #1("") -> (w822:string)
                    n246 = Concatenate Strings(w822, w818) -> (w823:string)
                    n247 = feedback-in #1(w823) -> ()
                    n248 = property on="read buffer" class="Str"("Value"=w823, "Text.Scroll Position"=w814) -> ()  [unwired: 2 in, 2 out]
                    "Horizontal Progress Bar" <- w815
                  }
                  n249 = VISA Flush I/O Buffer(VISA resource name=w791, error in (no error)=w793) -> (error out=w792:errorcluster)  [unwired: 1 in, 1 out]
                }
              }
              n250 = property on="Serial Monitor" class="Bool (strict)"(error in=w769) -> (error out=w768:errorcluster, "Value"=w770:bool)  [unwired: 1 in, 1 out]
              n251 = case shown="False" w770 {
                tunnel: w768 -> [w780 w781]
                tunnel: [w777 w781] -> w764
                frame False {
                  w776 = TRUE ("Visible")
                  n252 = property on="PlayPause Data Array" class="Bool (strict)"("Visible"=w776) -> ()  [unwired: 2 in, 2 out]
                  n253 = property on="read buffer" class="Str"(error in=w780, "Visible"=FALSE) -> (error out=w778:errorcluster)  [unwired: 1 in, 1 out]
                  n254 = property on="Clear Data Array" class="Bool (strict)"("Visible"=w776) -> ()  [unwired: 2 in, 2 out]
                  n255 = property on="CAN Data" class="Arr (strict)"(error in=w778, "Visible"=w776) -> (error out=w777:errorcluster)  [unwired: 1 in, 1 out]
                }
                frame True {
                }
              }
              n256 = call "Display Message to User5"("error in (no error)"=w764) -> ("error out"=w763:errorcluster)  [unwired: 9 in, 1 out]
            }
            event "Help Button": Value Change {
              n257 = event-data() -> ()  [unwired: 1 in, 6 out]
              n258 = control-ref of="This VI"() -> (w868:refnum<vi>)
              n259 = property class="VI"(reference=w868, error in=w866, "FP:Transparency"=u8 25 ("Front Panel Window:Transparency")) -> (reference out=w862:refnum<vi>, error out=w865:errorcluster)
              n260 = vi-ref "Help.vi"() -> (w872:refnum<vi>)
              n261 = invoke class="VI" method="FP.Open"(reference=w872, error in=w865, "Activate"=TRUE ("Activate?"), "State"=T13."Standard") -> (error out=w871:errorcluster)  [unwired: 1 in, 4 out]
              n262 = call "Help.vi"("error in"=w871, "TesterSWVersion"="1.7") -> ("error out"=w864:errorcluster)  [unwired: 6 in]
              n263 = property class="VI"(reference=w862, error in=w864, "FP:Transparency"=u8 0 ("Front Panel Window:Transparency")) -> (error out=w863:errorcluster)  [unwired: 1 out]
            }
            event "Can Send": Value Change {
              w907 = u8 0 items=["STATUS"=128, "EXTENDED"=2, "RTR"=1, "DATA MSG"=0] ("MSGTYPE")
              w912 = u8 1 items=["Standart flag", "Extern flag"] ("Format")
              w911 = u8 0 items=["Data flag", "Remote flag"] ("Type")
              # "Send"
              n264 = event-data() -> ()  [unwired: 1 in, 6 out]
              n265 = In Range and Coerce(upper limit=u16 18001, x="Motor Speed RPM", lower limit=u16 0) -> (coerced(x)=w894:u16, In Range?=w892:bool)
              n266 = In Range and Coerce(upper limit=u16 100, x="Motor Phase Current", lower limit=u16 40) -> (coerced(x)=w883:u16, In Range?=w885:bool)
              n267 = Not(x=w892) -> (.not. x?=w893:bool)
              n268 = Not(x=w885) -> (.not. x?=w884:bool)
              n269 = call "Display Message to User"("Enable"=w893) -> ()  [unwired: 9 in, 2 out]
              n270 = Select(t=w894, s=w892, f=u16 0) -> (s? t:f=w896:u16)
              n271 = call "Display Message to User6"("Enable"=w884) -> ()  [unwired: 9 in, 2 out]
              n272 = Select(t=w883, s=w885, f=u16 0) -> (s? t:f=w878:u16)
              n273 = property on="UUT" class="DigNum (strict)"() -> ("Value"=w890:u8)  [unwired: 2 in, 2 out]
              n274 = Split Number(x=w896) -> (hi(x)=w899:u8, lo(x)=w900:u8)
              n275 = case shown="79" w890 {
                tunnel: [u32 417357607 u32 417353582 u32 417349415 u32 417345319] -> w891
                frame 95, Default {
                }
                frame 79 {
                }
                frame 63 {
                }
                frame 47 {
                }
              }
              n276 = case shown="79" w890 {
                tunnel: [w931 w940 w953 w967] -> w905
                tunnel: w900 -> [w930 w939 w952 w966]
                tunnel: w899 -> [w929 w938 w951 w965]
                tunnel: "Motor Speed RPM" -> [w926 w935 _ _]
                tunnel: "Speed control" -> [_ _ w944 w958]
                tunnel: "Motor Over Temp" -> [_ _ w943 w957]
                tunnel: w878 -> [_ _ _ w954]
                frame 47, Default {
                  w928 = u8 0 ("element")
                  n277 = case shown="1, Default" w926 {
                    tunnel: [u8 1 ("element") u8 0 ("element")] -> w925
                    frame 1, Default {
                    }
                    frame 0 {
                    }
                  }
                  n278 = Build Array(u8 1 ("element"), w930, w929, w925, w928, w928, w928, w928) -> (w931:u8[])
                }
                frame 63 {
                  w936 = u8 0 ("element")
                  n279 = case shown="1, Default" w935 {
                    tunnel: [u8 1 ("element") u8 0 ("element")] -> w934
                    frame 1, Default {
                    }
                    frame 0 {
                    }
                  }
                  n280 = Build Array(u8 1 ("element"), w939, w938, w934, w936, w936, w936, w936) -> (w940:u8[])
                }
                frame 95 {
                  w949 = u8 0 ("element")
                  n281 = Boolean To (0,1)(Boolean=w944) -> (0, 1=w947:i16)
                  n282 = Boolean To (0,1)(Boolean=w943) -> (0, 1=w948:i16)
                  n283 = To Unsigned Byte Integer(number=w947) -> (unsigned 8bit integer=w946:u8)
                  n284 = To Unsigned Byte Integer(number=w948) -> (unsigned 8bit integer=w945:u8)
                  n285 = Build Array(u8 1 ("element"), w952, w951, w946, w945, w949, w949, w949) -> (w953:u8[])
                }
                frame 79 {
                  n286 = Split Number(x=w954) -> (hi(x)=w955:u8, lo(x)=w956:u8)
                  n287 = Boolean To (0,1)(Boolean=w958) -> (0, 1=w961:i16)
                  n288 = Boolean To (0,1)(Boolean=w957) -> (0, 1=w962:i16)
                  n289 = To Unsigned Byte Integer(number=w961) -> (unsigned 8bit integer=w960:u8)
                  n290 = To Unsigned Byte Integer(number=w962) -> (unsigned 8bit integer=w959:u8)
                  n291 = Build Array(u8 1 ("element"), w966, w965, w960, w959, w956, w955, u8 0 ("element")) -> (w967:u8[])
                }
              }
              n292 = Array Size(array=w905) -> (size(s)=w910:i32)
              n293 = call "Array Data to Single Num in Hex.vi"("aDATA"=w905) -> ("Numeric"=→"Data Send":u64)  [unwired: 10 in]
              n294 = To Unsigned Byte Integer(number=w910) -> (unsigned 8bit integer=w908:u8)
              n295 = call "CANAnalData.vi"("ID"=w891, "Data"=w905, "Config"=w903) -> ()  [unwired: 4 in, 5 out]
              n296 = Bundle By Name(cluster=T10 {"ID"=0, "MSGTYPE"=0, "LEN"=0, "aDATA"=[]} ("MsgTX 2"), "ID"=w891, "MSGTYPE"=w907, "LEN"=w908, "aDATA"=w905) -> (w906:T10)
              n297 = Unbundle By Name(w906) -> ("ID"=w920:u32, "LEN"=w921:u8, "aDATA"=w922:u8[])  [unwired: 1 out]
              n298 = property class="Clust (strict)"(reference=w903) -> ("Value"=w919:T8)  [unwired: 1 in, 2 out]
              n299 = Bundle By Name(cluster=T14 {"ID"=0, "TimeStamp"=0, "TimeFlag"=0, "SendType"=0, "RemoteFlag"=0, "ExternFlag"=0, "DataLen"=0, "Data"=[], "Reserved"=[]} ("Send"), "ID"=w920, "RemoteFlag"=w911, "ExternFlag"=w912, "DataLen"=w921, "Data"=w922) -> (w917:T14)
              n300 = Unbundle By Name(w919) -> ("DevType"=w913:T2, "DevIndex"=w914:u32, "CanIndex"=w915:T3)
              n301 = Build Array(w917) -> (w916:T14[])
              n302 = call "VCI_Transmit.vi"("Buffer"=w916, "CANIndex"=w915, "DevIndex"=w914, "DevType"=w913) -> ()  [unwired: 1 in, 7 out]
            }
            event "Graph Button": Value Change {
              w972 = FALSE ("Visible")
              n303 = event-data() -> ()  [unwired: 1 in, 6 out]
              n304 = Not(x="Graph Button") -> (.not. x?=w973:bool)
              n305 = property on="PlayPause Data Array" class="Bool (strict)"("Visible"=w973) -> ()  [unwired: 2 in, 2 out]
              n306 = property on="CAN Data" class="Arr (strict)"(error in=w974, "Visible"=w973) -> (error out=w975:errorcluster)  [unwired: 1 in, 1 out]
              n307 = property on="Clear Data Array" class="Bool (strict)"("Visible"=w973) -> ()  [unwired: 2 in, 2 out]
              n308 = property on="Waveform Chart" class="WFChart (strict)"(error in=w975, "Visible"="Graph Button") -> (error out=w977:errorcluster)  [unwired: 1 in, 1 out]
              n309 = property on="Serial Monitor" class="Bool (strict)"(error in=w977) -> (error out=w991:errorcluster, "Value"=w992:bool)  [unwired: 1 in, 1 out]
              n310 = case shown="True" w992 {
                tunnel: w991 -> [w999 w1004]
                tunnel: [w997 w1001] -> w980
                frame False {
                  n311 = property on="read buffer" class="Str"(error in=w999, "Visible"=FALSE) -> (error out=w997:errorcluster)  [unwired: 1 in, 1 out]
                }
                frame True {
                  w1000 = FALSE ("Visible")
                  n312 = property on="PlayPause Data Array" class="Bool (strict)"("Visible"=w1000) -> ()  [unwired: 2 in, 2 out]
                  n313 = property on="read buffer" class="Str"(error in=w1004, "Visible"=TRUE) -> (error out=w1002:errorcluster)  [unwired: 1 in, 1 out]
                  n314 = property on="Clear Data Array" class="Bool (strict)"("Visible"=w1000) -> ()  [unwired: 2 in, 2 out]
                  n315 = property on="CAN Data" class="Arr (strict)"(error in=w1002, "Visible"=w1000) -> (error out=w1001:errorcluster)  [unwired: 1 in, 1 out]
                }
              }
              n316 = property on="Serial Monitor" class="Bool (strict)"(error in=w980, "Value"=FALSE ("Serial Monitor")) -> (error out=w978:errorcluster)  [unwired: 1 in, 1 out]
              n317 = property on="Index" class="Ring (strict)"(error in=w978, "Visible"=w972) -> (error out=w988:errorcluster)  [unwired: 1 in, 1 out]
              n318 = property on="Value 1/2" class="Enum (strict)"(error in=w988, "Visible"=w972) -> (error out=w987:errorcluster)  [unwired: 1 in, 1 out]
              n319 = property on="Value" class="DigNum (strict)"(error in=w987, "Visible"=w972) -> (error out=w986:errorcluster)  [unwired: 1 in, 1 out]
              n320 = property on="SetGet" class="Enum (strict)"(error in=w986, "Visible"=w972) -> (error out=w985:errorcluster)  [unwired: 1 in, 1 out]
              n321 = property on="Serial Send" class="Bool (strict)"(error in=w985, "Visible"=w972) -> (error out=w983:errorcluster)  [unwired: 1 in, 1 out]
              n322 = property on="Clear Monitor" class="Bool"(error in=w983, "Visible"=w972) -> (error out=w982:errorcluster)  [unwired: 1 in, 1 out]
              n323 = property on="Function" class="Enum (strict)"(error in=w982, "Visible"=w972) -> (error out=w984:errorcluster)  [unwired: 1 in, 1 out]
              n324 = property on="Index" class="Ring (strict)"(error in=w984, "Visible"=w972) -> (error out=w989:errorcluster)  [unwired: 1 in, 1 out]
              n325 = property on="read buffer" class="Str"(error in=w989, "Visible"=w972) -> (error out=w981:errorcluster)  [unwired: 1 in, 1 out]
            }
            event "Serial Com": Value Change {
              n326 = event-data() -> ()  [unwired: 1 in, 6 out]
              n327 = property on="Serial Com" class="Bool"(error in=w1009, "Visible"=FALSE) -> (error out=w1008:errorcluster)  [unwired: 1 in, 1 out]
              n328 = property on="VISA resource name" class="VISAName"(error in=w1008, "Visible"=TRUE) -> (error out=w1006:errorcluster)  [unwired: 1 in, 1 out]
            }
            event "VISA resource name": Value Change {
              n329 = event-data() -> ()  [unwired: 1 in, 1 out]
              n330 = control-ref of="This VI"() -> (w1015:refnum<vi>)
              n331 = call "Serial InitMarvin.vi"("error in (no error)"=w1024, "VI reference (current VI)"=w1015, "VISA Refnum in"="VISA resource name") -> ("error out"=w1033:errorcluster, "Boolean"=w1021:bool)  [unwired: 7 in]
              n332 = property on="Serial Status" class="Bool (strict)"(error in=w1033, "Value"=w1021) -> (error out=w1027:errorcluster)  [unwired: 1 in, 1 out]
              n333 = property on="VISA resource name" class="VISAName"(error in=w1027, "Visible"=FALSE) -> (error out=w1026:errorcluster)  [unwired: 1 in, 1 out]
              n334 = property on="Serial Com" class="Bool"(error in=w1026, "Visible"=TRUE) -> (error out=w1019:errorcluster)  [unwired: 1 in, 1 out]
              n335 = call "Serial.vi"("error in (no error)"=w1019, "Clear Log"=TRUE, "VISA resource name"="VISA resource name") -> ("error out"=w1017:errorcluster)  [unwired: 7 in, 1 out]
              n336 = call <vilib>:"Clear Errors.vi"("error in (no error)"=w1017) -> ("error out"=w1023:errorcluster)  [unwired: 5 in, 1 out]
              n337 = case shown="True" w1021 {
                tunnel: w1023 -> [w1034 w1037]
                tunnel: [w1034 w1036] -> w1022
                tunnel: "VISA resource name" -> [_ w1035]
                frame False {
                }
                frame True {
                  n338 = VISA Flush I/O Buffer(VISA resource name=w1035, error in (no error)=w1037) -> (error out=w1036:errorcluster)  [unwired: 1 in, 1 out]
                }
              }
            }
            event "Stop": Value Change {
              n339 = event-data() -> ()  [unwired: 1 in, 6 out]
              n340 = Flush Queue(queue=w1043, error in (no error)=w1042) -> (queue out=w1041:refnum<queue>, error out=w1040:errorcluster)  [unwired: 1 out]
              n341 = Release Queue(queue=w1041, error in (no error)=w1040) -> (error out=w1039:errorcluster)  [unwired: 1 in, 2 out]
            }
            event "Refresh Button": Value Change {
              n342 = event-data() -> ()  [unwired: 1 in, 6 out]
              n343 = Release Queue(queue=w1049, error in (no error)=w1050) -> (error out=w1048:errorcluster)  [unwired: 1 in, 2 out]
            }
          }
          n344 = Unbundle By Name(w330) -> ("status"=w336:bool)
          n345 = Or(x=w336, y=w328) -> (x .or. y?=w335:bool)
        }
        n346 = while {
          shift-right: [w149] -> _
          shift-left: w119 -> [w151]
          shift-right: [w147] -> _
          shift-left: _ -> [w148]
          shift-right: [w143] -> _
          shift-left: w118 -> [w143]
          shift-right: [w141] -> w115
          shift-left: w109 -> [w136]
          shift-right: [w135] -> w114
          shift-left: w108 -> [w142]
          shift-right: [w134] -> w113
          shift-left: w107 -> [w140]
          shift-right: [w133] -> w112
          shift-left: w106 -> [w139]
          shift-right: [w138] -> w110
          shift-left: w111 -> [w137]
          shift-right: [w126] -> _
          shift-left: cluster{"Frame Data":u64, "Frame ID":u32}[] [] ("Array 3") -> [w128]
          stop <- w150 stop-if-true
          n347 = Dequeue Element(queue=w151, error in (no error)=w143) -> (queue out=w149:refnum<queue>, element=w144:T9, error out=w150:errorcluster)  [unwired: 1 in, 1 out]
          n348 = for {
            tunnel: [w314] -> w146 mode=indexing
            tunnel: w144 -> [w316] mode=indexing
            tunnel: [w315] -> w145 mode=indexing
            tunnel: [w313] -> w132 mode=indexing
            tunnel: [w312] -> w131 mode=indexing
            shift-right: [w312] -> _
            shift-left: _ -> [w311]
            n349 = Unbundle By Name(w316) -> ("ID"=w313:u32, "aDATA"=w315:u8[])
            n350 = call "Array Data to Single Num in Hex.vi"("aDATA"=w315) -> ("Numeric"=w314:u64)  [unwired: 10 in]
            n351 = case shown="Default" w313 {
              tunnel: w314 -> [_ w321]
              tunnel: w313 -> [_ w320]
              tunnel: [w317 w319] -> w312
              tunnel: w311 -> [w317 _]
              frame 0 {
              }
              frame Default {
                n352 = Bundle By Name(cluster=cluster{"Frame Data":u64, "Frame ID":u32} {"Frame Data"=0, "Frame ID"=0} ("Cluster"), "Frame ID"=w320, "Frame Data"=w321) -> (w319:cluster{"Frame Data":u64, "Frame ID":u32})
              }
            }
          }
          n353 = case shown="True" "PlayPause Data Array" {
            tunnel: w131 -> [w154 _]
            tunnel: w128 -> [w153 w155]
            tunnel: [w152 w155] -> w127
            frame False {
              n354 = Build Array (concatenate)(w154, w153) -> (w152:cluster{"Frame Data":u64, "Frame ID":u32}[])
            }
            frame True {
            }
          }
          n355 = Build Array (concatenate)(w146, w148) -> (w147:u64[][])
          "Array" <- w147
          n356 = Select(t=cluster{"Frame Data":u64, "Frame ID":u32}[] [], s="Clear Data Array", f=w127) -> (s? t:f=w126:cluster{"Frame Data":u64, "Frame ID":u32}[])
          "CAN Data" <- w126
          n357 = for {
            tunnel: w145 -> [w167] mode=indexing
            tunnel: [w162] -> w138
            tunnel: w137 -> [w161]
            shift-right: [w165] -> w141
            shift-left: w136 -> [w160]
            shift-right: [w159] -> w135
            shift-left: w142 -> [w166]
            shift-right: [w158] -> w134
            shift-left: w140 -> [w164]
            shift-right: [w157] -> w133
            shift-left: w139 -> [w163]
            tunnel: w132 -> [w156] mode=indexing
            n358 = case shown="417539903, 417539919, 417539935" w156 {
              tunnel: w167 -> [_ w210 w257 w310]
              tunnel: w160 -> [w171 w186 w248 w301]
              tunnel: w166 -> [w170 w185 w247 w300]
              tunnel: [w171 w176 w248 w301] -> w165
              tunnel: [w170 w182 w247 w300] -> w159
              tunnel: [w169 w181 w246 w299] -> w158
              tunnel: w164 -> [w169 w180 w246 w299]
              tunnel: [w168 w177 w245 w287] -> w157
              tunnel: w163 -> [w168 w177 w245 _]
              tunnel: [w172 w175 w244 w298] -> w162
              tunnel: w161 -> [w172 w174 w244 w298]
              frame Default {
              }
              frame 417408831, 417408847, 417408863 {
                # "Frame ID\n0x18E1273F"
                n359 = Index Array(array=w210, index #1=0 ("index"), index #2=1 ("index"), index #3=2 ("index"), index #4=3 ("index"), index #5=4 ("index"), index #6=5 ("index"), index #7=6 ("index"), index #8=7 ("index")) -> (element #1=w194:u8, element #2=w196:u8, element #3=w197:u8, element #4=w201:u8, element #5=w204:u8, element #6=w208:u8, element #7=w209:u8, element #8=w207:u8)
                n360 = Join Numbers(hi=w209, lo=w208) -> ((hi.lo)=w228:u16)
                n361 = Join Numbers(hi=w197, lo=w196) -> ((hi.lo)=w198:u16)
                n362 = Number To Hexadecimal String(2:w228) -> (0:w227:string)  [unwired: 1 in]
                n363 = Number To Hexadecimal String(2:w207) -> (0:w221:string)  [unwired: 1 in]
                n364 = Number To Hexadecimal String(2:w194) -> (0:w195:string)  [unwired: 1 in]
                n365 = Number To Hexadecimal String(2:w198) -> (0:w199:string)  [unwired: 1 in]
                n366 = Number To Hexadecimal String(2:w201) -> (0:w202:string)  [unwired: 1 in]
                n367 = Number To Hexadecimal String(2:w204) -> (0:w205:string)  [unwired: 1 in]
                n368 = Hexadecimal String To Number(string=w195) -> (number=w192:u32)  [unwired: 2 in, 1 out]
                n369 = Hexadecimal String To Number(string=w199) -> (number=w200:u32)  [unwired: 2 in, 1 out]
                n370 = Hexadecimal String To Number(string=w202) -> (number=w203:u32)  [unwired: 2 in, 1 out]
                n371 = Hexadecimal String To Number(string=w205) -> (number=w206:u32)  [unwired: 2 in, 1 out]
                n372 = Hexadecimal String To Number(string=w221) -> (number=w220:u32)  [unwired: 2 in, 1 out]
                n373 = Hexadecimal String To Number(string=w227) -> (number=w226:u32)  [unwired: 2 in, 1 out]
                n374 = To Unsigned Word Integer(number=w192) -> (unsigned 16bit integer=→"ECS State":u16)
                n375 = To Double Precision Float(number=w200) -> (double precision float=w187:dbl)
                n376 = To Double Precision Float(number=w226) -> (double precision float=w223:dbl)
                n377 = To Double Precision Float(number=w220) -> (double precision float=→"DC Current":dbl)
                n378 = To Double Precision Float(number=w203) -> (double precision float=w191:dbl)
                n379 = To Double Precision Float(number=w206) -> (double precision float=w189:dbl)
                n380 = To Double Precision Float(number=u32 10 ("y")) -> (double precision float=w224:dbl)
                n381 = Subtract(x=w189, y=50.0 ("x")) -> (x-y=w179:dbl)
                n382 = Subtract(x=w191, y=50.0 ("x")) -> (x-y=w184:dbl)
                n383 = disable-structure shown="Enabled" {
                  disable-tunnel: w187 -> [w232 w233]
                  disable-tunnel: w186 -> [w231 _]
                  disable-tunnel: [w229 w233] -> w176
                  frame Disabled {
                    n384 = call "Filter (SubVI).vi"("Delta"=3500.0, "NewVal"=w232, "OldVal"=w231) -> ("Val"=w229:dbl)  [unwired: 8 in]
                  }
                  frame Enabled {
                  }
                }
                "Motor Speed RPM" <- w176
                n385 = Divide(x=w223, y=w224) -> (x/y=→"DC Voltage":dbl)
                n386 = call "Filter (SubVI).vi"("Delta"=100.0, "NewVal"=w179, "OldVal"=w180) -> ("Val"=w181:dbl)  [unwired: 8 in]
                "Power transistor Heat sink Temp." <- w181
                n387 = call "Filter (SubVI).vi"("Delta"=130.0, "NewVal"=w184, "OldVal"=w185) -> ("Val"=w182:dbl)  [unwired: 8 in]
                "Motor Stator Temp." <- w182
                n388 = case shown="True" TRUE {
                  tunnel: w174 -> [w234 w237]
                  tunnel: [w234 w236] -> w175
                  tunnel: w176 -> [_ w235]
                  frame False {
                  }
                  frame True {
                    n389 = disable-structure shown="Disabled" {
                      disable-tunnel: w235 -> [w241 _]
                      frame Disabled {
                        n390 = call <vilib>:"Application Directory.vi"() -> ("Application Directory"=w239:path)
                        n391 = Build Path(base path=w239, name or relative path="RPM Log.lvm") -> (appended path=w240:path)
                        n392 = call "Write To Measurement File"("Signals"=w241, "Filename"=w240) -> ()  [unwired: 15 in, 3 out]
                      }
                      frame Enabled {
                      }
                    }
                    n393 = Build Array (concatenate)(w235, w237) -> (w236:dbl[])
                    "Waveform Chart" <- w236
                  }
                }
              }
              frame 417539903, 417539919, 417539935 {
                # "Framde ID\n0x18E3273F"
                n394 = property on="UUT" class="DigNum (strict)"() -> ("Value"=w243:u8)  [unwired: 2 in, 2 out]
                n395 = Index Array(array=w257, index #1=0 ("index"), index #2=1 ("index")) -> (element #1=w255:u8, element #2=w250:u8)
                n396 = case shown="Default" w243 {
                  tunnel: [0 1 2] -> w242
                  frame Default {
                  }
                  frame 95 {
                  }
                  frame 79 {
                  }
                }
                n397 = Number To Boolean Array(number=w255) -> (Boolean array=w254:bool[])
                n398 = Number To Boolean Array(number=w250) -> (Boolean array=w252:bool[])
                n399 = Boolean To (0,1)(Boolean=w252) -> (0, 1=w249:i16[])
                n400 = Boolean To (0,1)(Boolean=w254) -> (0, 1=w253:i16[])
                n401 = case shown="79, 95" w243 {
                  tunnel: w249 -> [_ w262]
                  tunnel: w242 -> [_ w261]
                  frame 0, Default {
                  }
                  frame 79, 95 {
                    n402 = for {
                      tunnel: w262 -> [w267] mode=indexing
                      tunnel: w261 -> [w263]
                      i -> [w264]
                      stop <- w265 stop-if-true
                      n403 = Not Equal To 0?(x=w267) -> (x != 0?=w266:bool)
                      n404 = case shown="2" w264 {
                        tunnel: w266 -> [w268 w269 w270]
                        frame 0, Default {
                          "Ambient Sensor temp" <- w268
                        }
                        frame 1 {
                          "Ambient Over temp" <- w269
                        }
                        frame 2 {
                          "Hall Sensor Fault" <- w270
                        }
                      }
                      n405 = Equal?(x=w264, y=w263) -> (x = y?=w265:bool)
                    }
                  }
                }
                n406 = for {
                  tunnel: w253 -> [w272] mode=indexing
                  i -> [w273]
                  n407 = Not Equal To 0?(x=w272) -> (x != 0?=w271:bool)
                  n408 = case shown="0, Default" w273 {
                    tunnel: w271 -> [w274 w275 w276 w277 w278 w279 w280 w281]
                    frame 0, Default {
                      "Drive Sensor temp Failure" <- w274
                    }
                    frame 1 {
                      "Drive Over temperature" <- w275
                    }
                    frame 2 {
                      "Motor Sensor temp Fauilre" <- w276
                    }
                    frame 3 {
                      "Motor Over temperature" <- w277
                    }
                    frame 4 {
                      "Derated drive temp" <- w278
                    }
                    frame 5 {
                      "Under voltage/Over voltage" <- w279
                    }
                    frame 6 {
                      "Commutation err" <- w280
                    }
                    frame 7 {
                      "Speed error" <- w281
                    }
                  }
                }
              }
              frame 417474367, 417474383, 417474399 {
                w289 = "."
                # "Frame ID\n0x18E2273F"
                n409 = Index Array(array=w310, index #1=0 ("index")) -> (element #1=w308:u8, element #2=w306:u8, element #3=w283:u8, element #4=w284:u8, element #5=w285:u8, element #6=w286:u8)  [unwired: 5 in]
                n410 = Split Number(x=w285) -> (hi(x)=w297:u8, lo(x)=w296:u8)
                n411 = Split Number(x=w286) -> (hi(x)=w295:u8, lo(x)=w294:u8)
                n412 = Join Numbers(hi=w284, lo=w283) -> ((hi.lo)=→"Motor Phase Current":u16)
                n413 = Number To Decimal String(number=w297) -> (decimal integer string=w293:string)  [unwired: 1 in]
                n414 = Number To Decimal String(number=w296) -> (decimal integer string=w292:string)  [unwired: 1 in]
                n415 = Number To Decimal String(number=w295) -> (decimal integer string=w291:string)  [unwired: 1 in]
                n416 = Number To Decimal String(number=w294) -> (decimal integer string=w290:string)  [unwired: 1 in]
                n417 = Concatenate Strings(w293, w289, w292, w289, w291, w289, w290) -> (→"Driver Version":string)
                n418 = Number To Hexadecimal String(2:w306) -> (0:w304:string)  [unwired: 1 in]
                n419 = Hexadecimal String To Number(string=w304) -> (number=w305:u32)  [unwired: 2 in, 1 out]
                n420 = To Double Precision Float(number=w305) -> (double precision float=w303:dbl)
                n421 = Subtract(x=w303, y=50.0) -> (x-y=w287:dbl)
                "Ambient Temperature" <- w287
                n422 = To Double Precision Float(number=w308) -> (double precision float=→"Motor Phase Current RMS":dbl)
              }
            }
          }
        }
      }
      frame "Stop" {
        n423 = Release Queue(queue=w1062, error in (no error)=w1064) -> (error out=w1063:errorcluster)  [unwired: 1 in, 2 out]
        n424 = flat-sequence {
          tunnel: w1061 -> [w1065]
          tunnel: [TRUE ("Stop")] -> w1060
          frame #0 {
            w1071 = u8[] [1, 0, 0, 0, 0, 0, 0, 0] ("Data 2")
            w1073 = u8 0 items=["STATUS"=128, "EXTENDED"=2, "RTR"=1, "DATA MSG"=0] ("MSGTYPE")
            w1078 = u8 1 items=["Standart flag", "Extern flag"] ("Format")
            w1077 = u8 0 items=["Data flag", "Remote flag"] ("Type")
            n425 = property on="Serial Status" class="Bool (strict)"() -> ("Value"=w1066:bool)  [unwired: 2 in, 2 out]
            n426 = property on="UUT" class="DigNum (strict)"() -> ("Value"=w1068:u8)  [unwired: 2 in, 2 out]
            n427 = case shown="True" w1066 {
              frame False {
              }
              frame True {
                n428 = property on="VISA resource name" class="VISAName"() -> ("Value"=w1089:refnum<visa-resource-name>)  [unwired: 2 in, 2 out]
                n429 = VISA Close(VISA resource name=w1089) -> ()  [unwired: 1 in, 1 out]
              }
            }
            n430 = case shown="95, Default" w1068 {
              tunnel: [u32 417357607 u32 417349415 u32 417345319] -> w1067
              frame 95, Default {
              }
              frame 63 {
              }
              frame 47 {
              }
            }
            n431 = property on="Graph Button" class="Bool (strict)"("Value"=FALSE ("Graph Button")) -> ()  [unwired: 2 in, 2 out]
            n432 = Array Size(array=w1071) -> (size(s)=w1076:i32)
            n433 = To Unsigned Byte Integer(number=w1076) -> (unsigned 8bit integer=w1074:u8)
            n434 = Bundle By Name(cluster=T10 {"ID"=0, "MSGTYPE"=0, "LEN"=0, "aDATA"=[]} ("MsgTX 2"), "ID"=w1067, "MSGTYPE"=w1073, "LEN"=w1074, "aDATA"=w1071) -> (w1072:T10)
            n435 = call "CANAnalData.vi"("ID"=w1067, "Data"=w1071, "Config"=w1065) -> ()  [unwired: 4 in, 5 out]
            n436 = call "Array Data to Single Num in Hex.vi"("aDATA"=w1071) -> ("Numeric"=w1070:u64)  [unwired: 10 in]
            n437 = property on="Data Send" class="DigNum (strict)"("Value"=w1070) -> ()  [unwired: 2 in, 2 out]
            n438 = Unbundle By Name(w1072) -> ("ID"=w1086:u32, "LEN"=w1087:u8, "aDATA"=w1088:u8[])  [unwired: 1 out]
            n439 = property class="Clust (strict)"(reference=w1065) -> ("Value"=w1085:T8)  [unwired: 1 in, 2 out]
            n440 = Bundle By Name(cluster=T14 {"ID"=0, "TimeStamp"=0, "TimeFlag"=0, "SendType"=0, "RemoteFlag"=0, "ExternFlag"=0, "DataLen"=0, "Data"=[], "Reserved"=[]} ("Send"), "ID"=w1086, "RemoteFlag"=w1077, "ExternFlag"=w1078, "DataLen"=w1087, "Data"=w1088) -> (w1083:T14)
            n441 = Unbundle By Name(w1085) -> ("DevType"=w1079:T2, "DevIndex"=w1080:u32, "CanIndex"=w1081:T3)
            n442 = Build Array(w1083) -> (w1082:T14[])
            n443 = call "VCI_Transmit.vi"("Buffer"=w1082, "CANIndex"=w1081, "DevIndex"=w1080, "DevType"=w1079) -> ()  [unwired: 1 in, 7 out]
          }
          frame #1 {
          }
        }
      }
    }
  }
  n444 = disable-structure shown="Disabled" {
    frame Disabled {
      n445 = control-ref of="Config_CANAT"() -> ()  [unwired: 1 out]
      n446 = control-ref of="UUT"() -> ()  [unwired: 1 out]
    }
    frame Enabled {
    }
  }
